vi "Interfaz_Completa.vi"() -> ()   [LabVIEW 2019]
panel:
  out "Datos UART":string
  in  "Nombre .csv":string
  in  "Export Button":bool
  out "UART Error":errorcluster
  out "Valores Tácteles":dbl[][](array[numeric])
  in  "Fila":i32
  in  "Columna":i32
  in  "Selección Modo Datos":T1(ring) caption="Modo Introducción de Datos"
  out "XY Graph":cluster{"Y":dbl[], "Y":dbl[]}[](graph)
  out "Intensity Graph":dbl[][](graph)
  in  "Tab_Introducción_Datos":T2(tab)
  in  "Comando Manual":bool
  in  "Cadena de datos (Manual)":string
  in  "Presión Manual(PSI)":dbl
  in  "Recibir de fichero":bool
  in  "file path (use dialog)":path
  in  "Nº De Ejecuciones":dbl
  in  "Tiempo Entre Medidas(ms)":dbl
  in  "Incremento":dbl
  in  "Presión Min (PSI)":dbl
  in  "Presión Max (PSI)":dbl
  in  "Tiempo Entre Medida(ms)":dbl
  in  "Tiempo Total":dbl
  in  "Presión Deseada (PSI)":dbl
  in  "Histéresis":bool
  in  "Deriva":bool
  in  "Medida Simple":bool
  in  "Tab_Valvula":enum32{"Page 2"}(tab)
  in  "Ejecutar Válvula":bool
  in  "Tipo de Comando":string(combo)
  in  "COM Pneumax":refnum<visa-resource-name>
  in  "Presión Deseada (PSI)":u8 step=5
  in  "Parámetro":u8 step=1
  in  "Valor del Parámetro":u8 max=25 step=1
  out "Presión (PSI)":dbl
  out "Respuesta del regulador":string
  in  "Nombre Nueva Sesión":string
  in  "Tab Control":enum32{"Tab_Automatica", "Tab_Manual"}(tab)
  in  "OK_Automatico":bool
  in  "baud rate PSoC":u32(ring)=9600 items=["75"=75, "110"=110, "134"=134, "150"=150, "300"=300, "600"=600, "1200"=1200, "1800"=1800, "2400"=2400, "4800"=4800, "7200"=7200, "9600"=9600, "14400"=14400, "19200"=19200, "28800"=28800, "38400"=38400, "56000"=56000, "57600"=57600, "115200"=115200, "128000"=128000, "230400"=230400]
  in  "COM PSoC":refnum<visa-resource-name>
  in  "OK_Manual":bool
  in  "NºFilas":i32
  in  "Nº Columnas":i32
  in  "N_Bits":i32
  in  "Proporcional":i32
  in  "Valor_Maximo":i32
  in  "Manual":bool
  in  "Automática":bool
  in  "Plantilla Tácteles":bool[][](array[boolean])
  in  "Home Button":bool
  in  "Sesiones Disponibles":u16(ring) items=["Default", "Prueba1", "Prueba8", "Prueba7", "Manu", "Andres"]
  in  "Stop Button":bool
  in  "Settings Button":bool
  in  "Save Button":bool
  in  "Refresh Button":bool
  in  "Open Button":bool
  # "Fila y Columna del Táctel a Representar"
  # "Abra el fichero que contiene los datos en el formato adecuado y pulse el botón inferior para leer una medida."
  # "Control de Electroválvula Pneumax"
  # "Configure los indicadores del modo Automático. Una vez haya realizado la\nconfiguración, pulse OK."
  # "Configure el número de filas y de columnas, si la medida viene de manera\n proporcional, el Nº de bits que tiene el timer con el que se ha realizado \nla medida y el valor máximo de las medidas. Luego pulse el botón OK y\n coloque los sensores que desee en su plantilla tácteles."
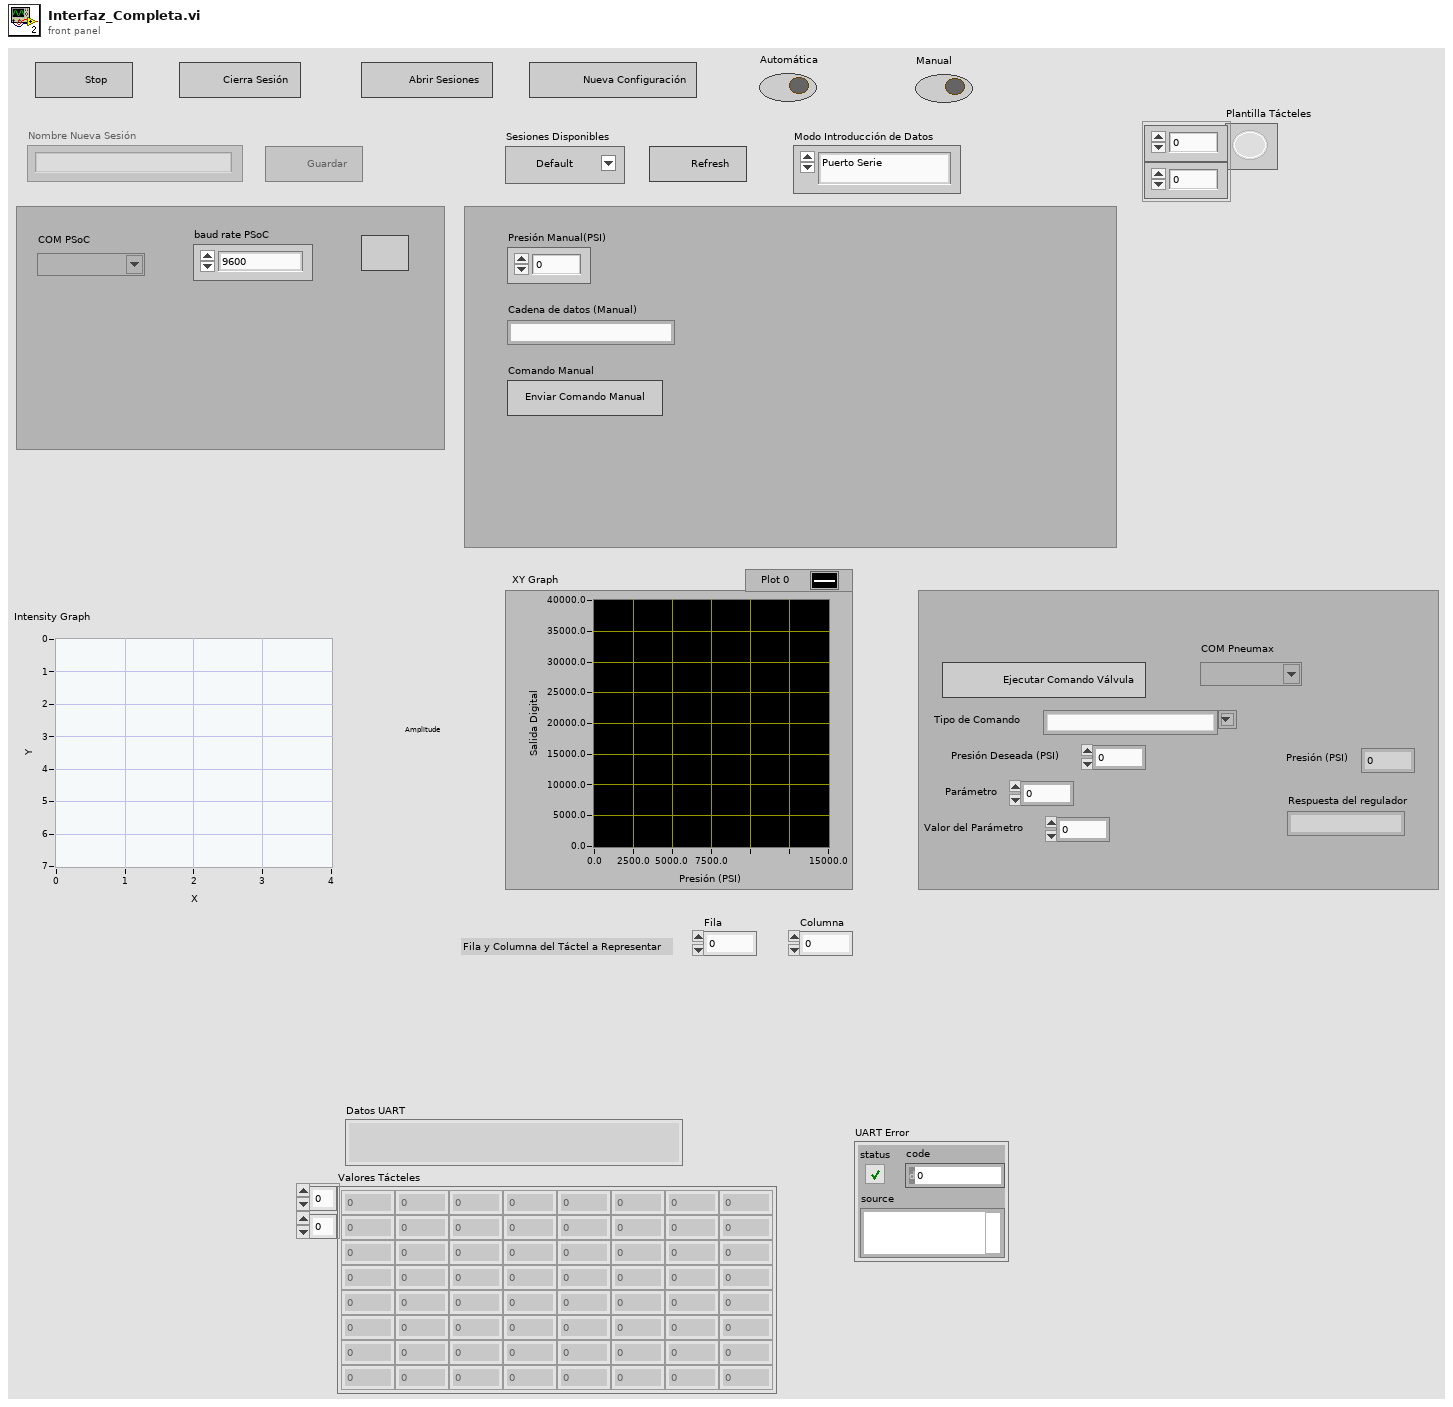
[diagram p1: front panel]
types:
  T1 = enum16{"Puerto Serie", "Archivo Importado", "Manual"}
  T2 = enum32{"Manual", "Archivo Importado", "Puerto Serie"}
  T3 = enum8{"Enabled", "Disabled", "Disabled and Grayed Out"}
  T4 = cluster{"String":string, i32, i32, i32, i32, i32}
  T5 = cluster{"Filas ":i32, "Columnas":i32, "Tacteles_Activados":bool[][]}
  T6 = cluster{"Value":string, "String_Tácteles":string, "Number of Rows":u32, "Number of Columns":u32, "Value":i32, "Value":i32, "Value":i32}
  T7 = cluster{"Value":refnum<visa-resource-name>, "Value":u32, "Value":refnum<visa-resource-name>, "Value":i32, "Value":i32}
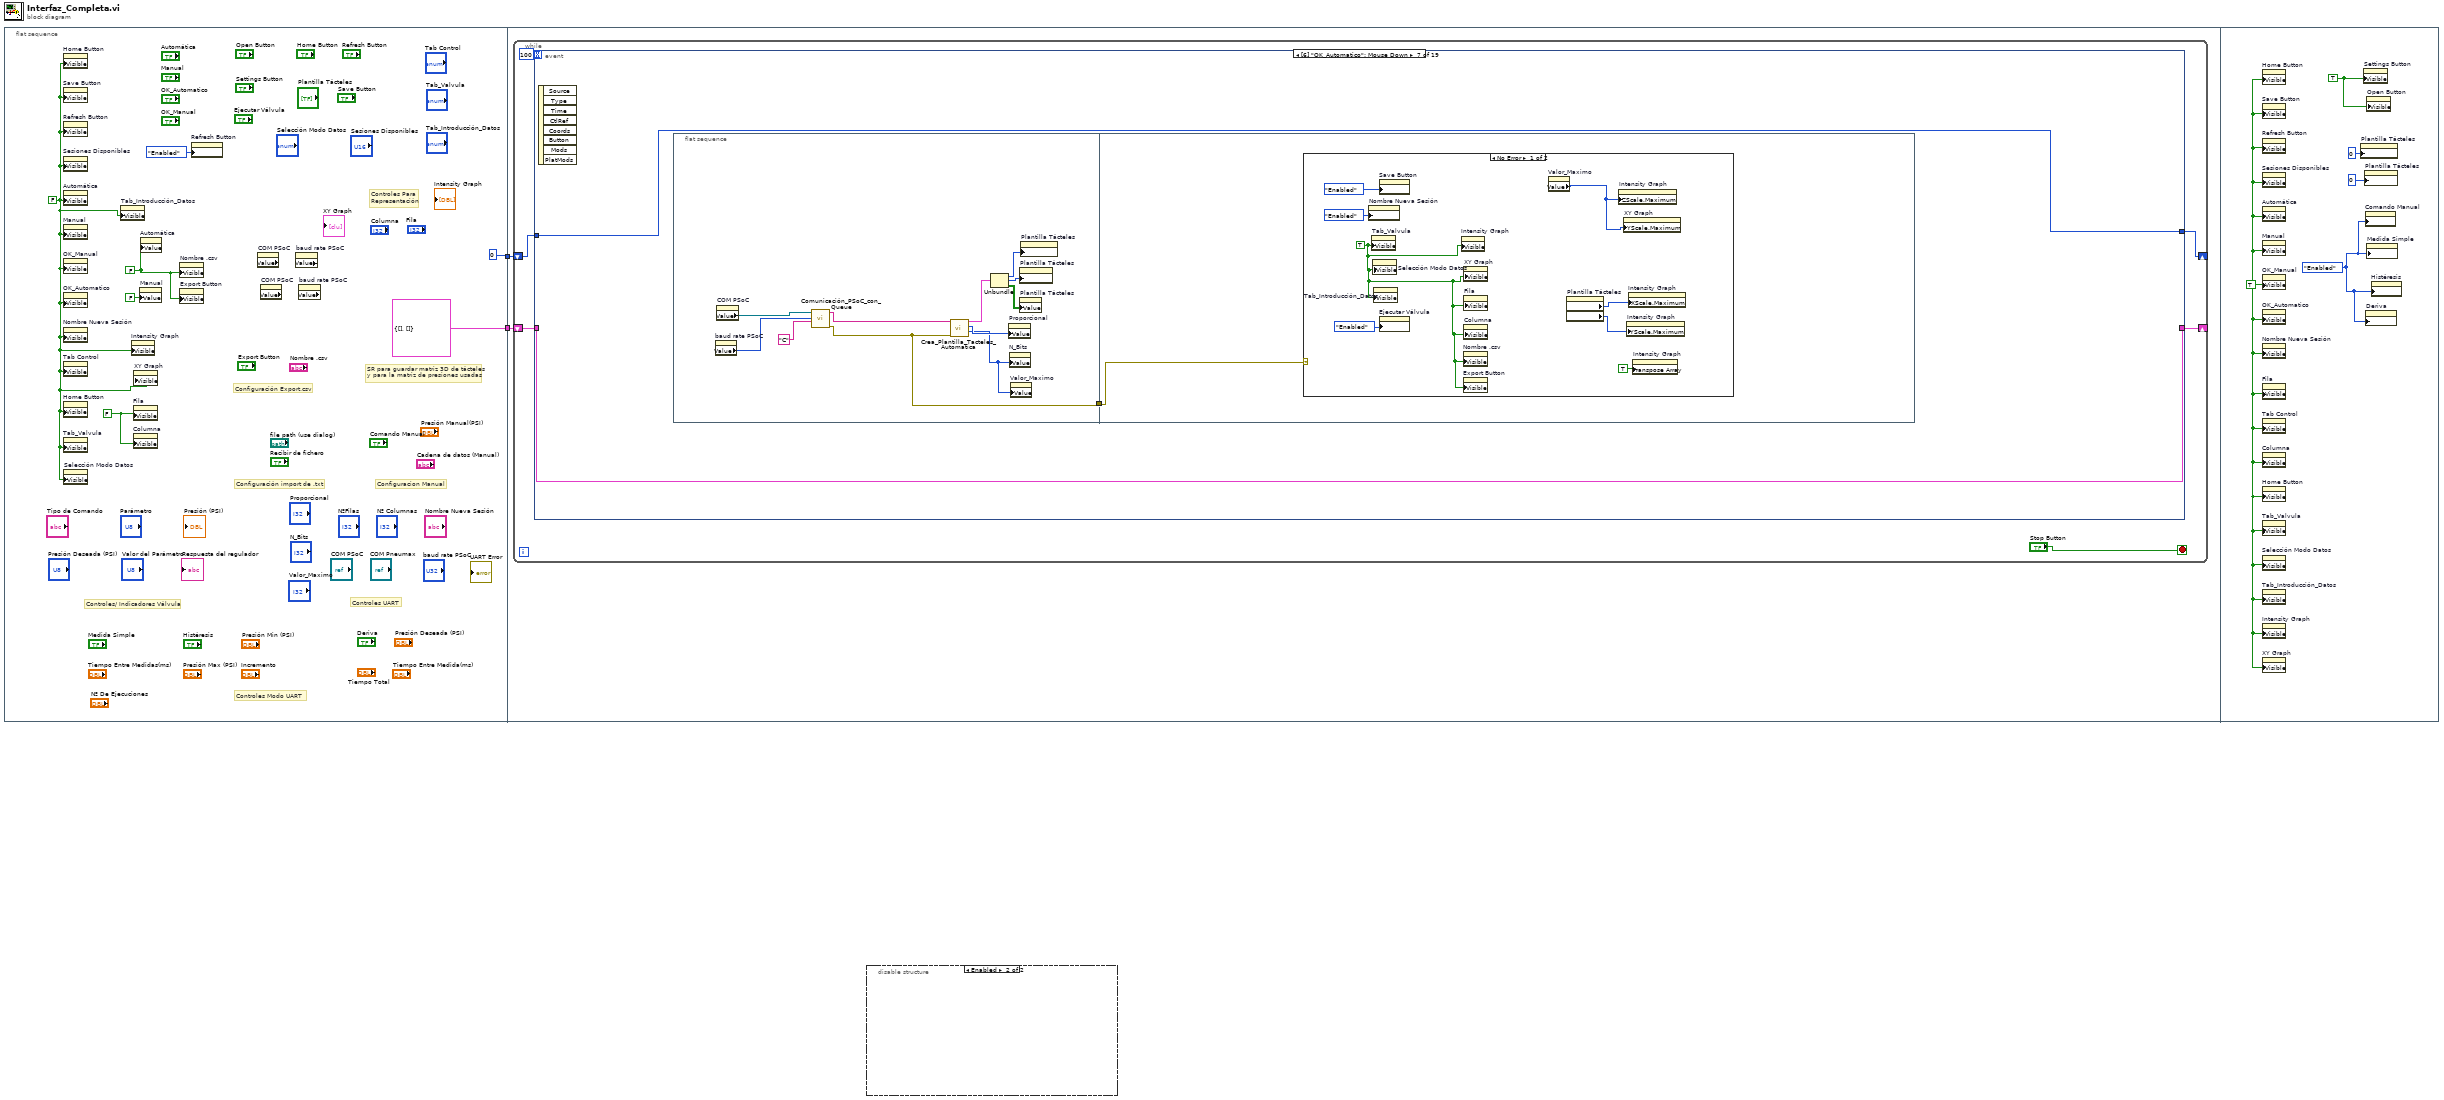
[diagram p0: block diagram]
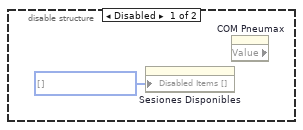
[diagram p2: hidden frame]
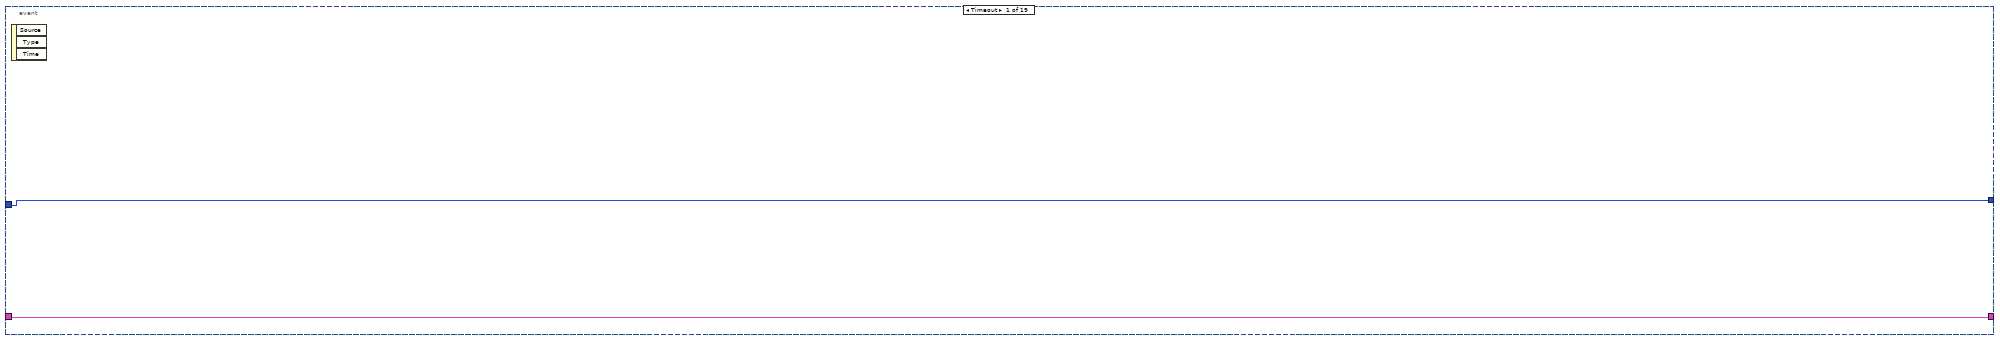
[diagram p3: hidden frame]
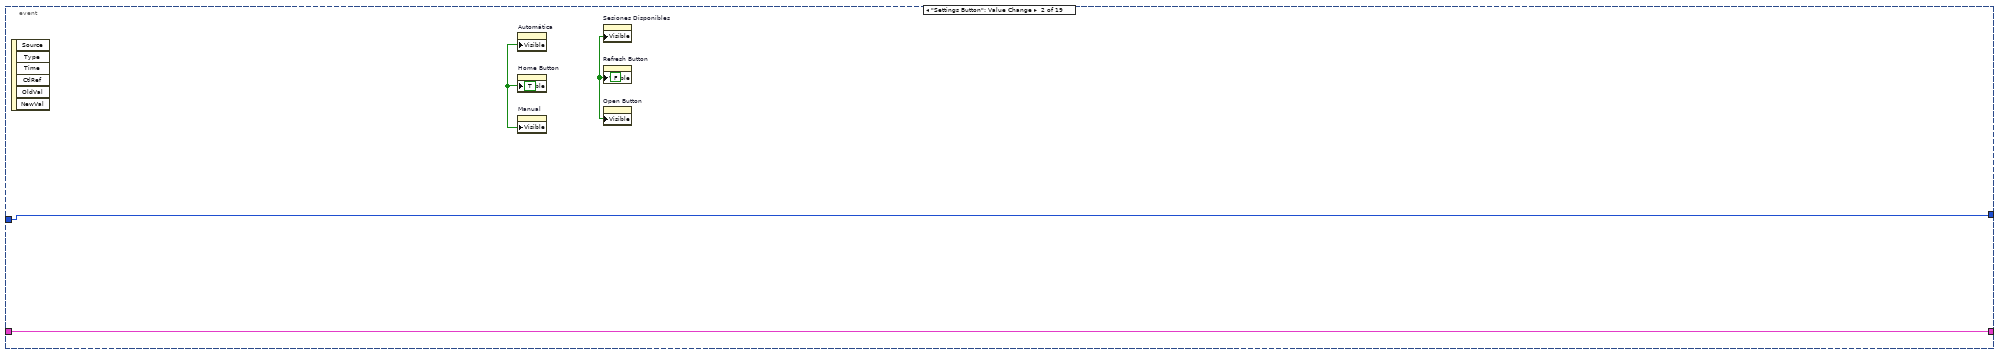
[diagram p4: hidden frame]
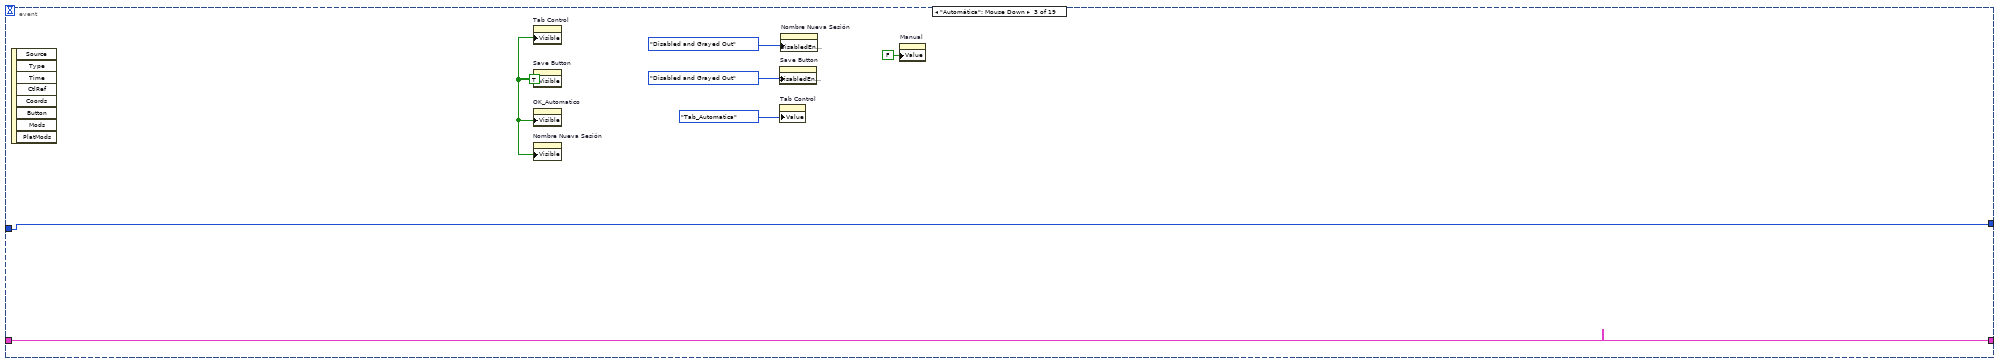
[diagram p5: hidden frame]
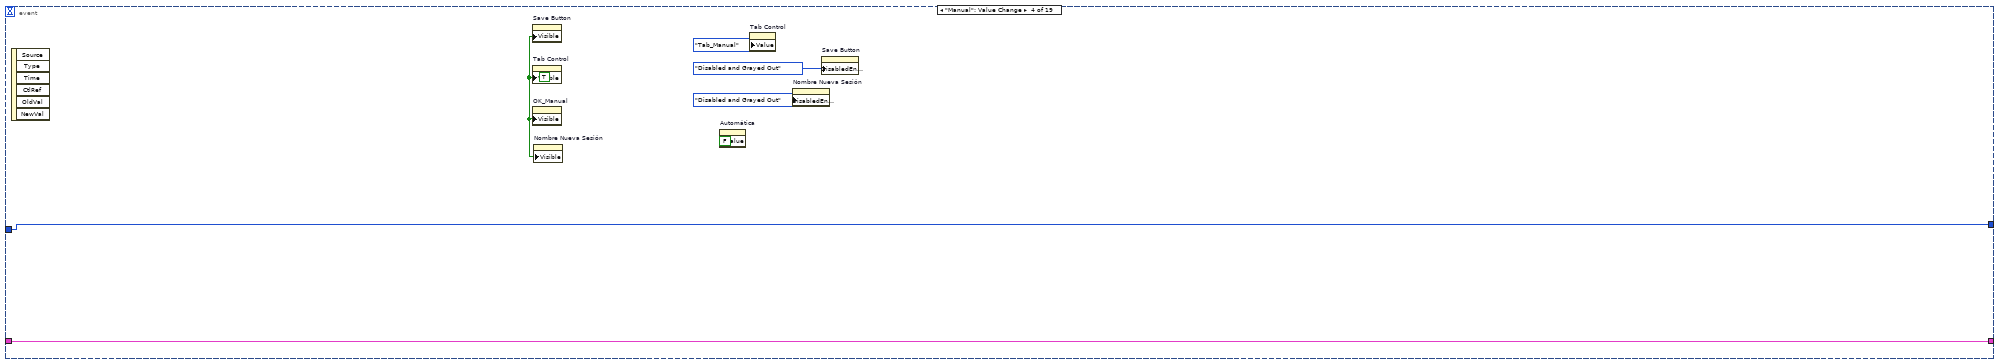
[diagram p6: hidden frame]
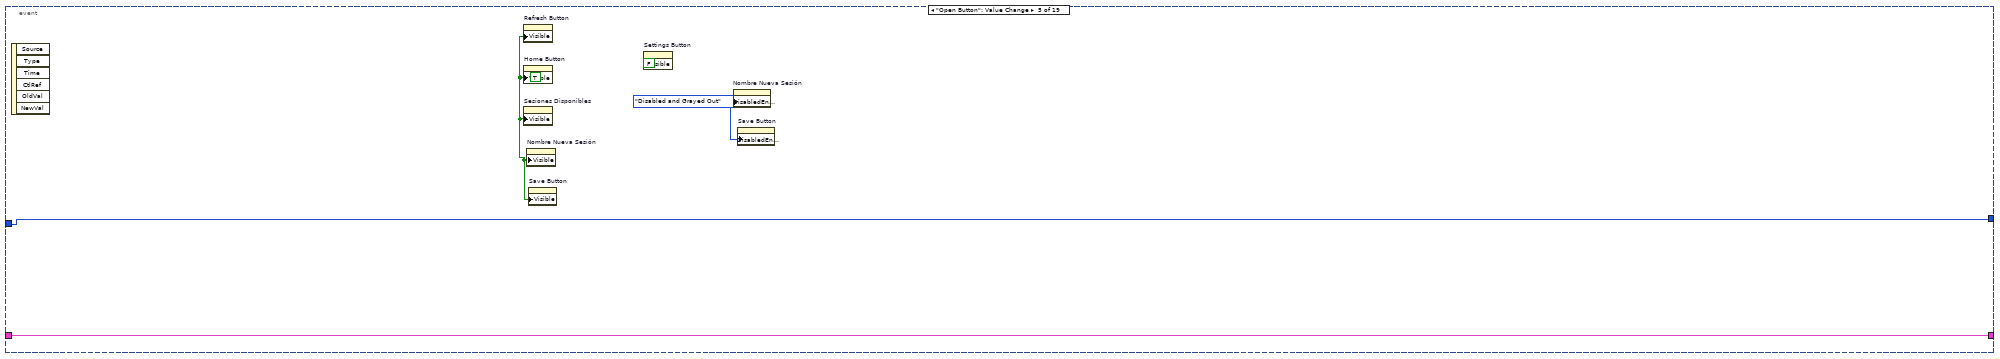
[diagram p7: hidden frame]
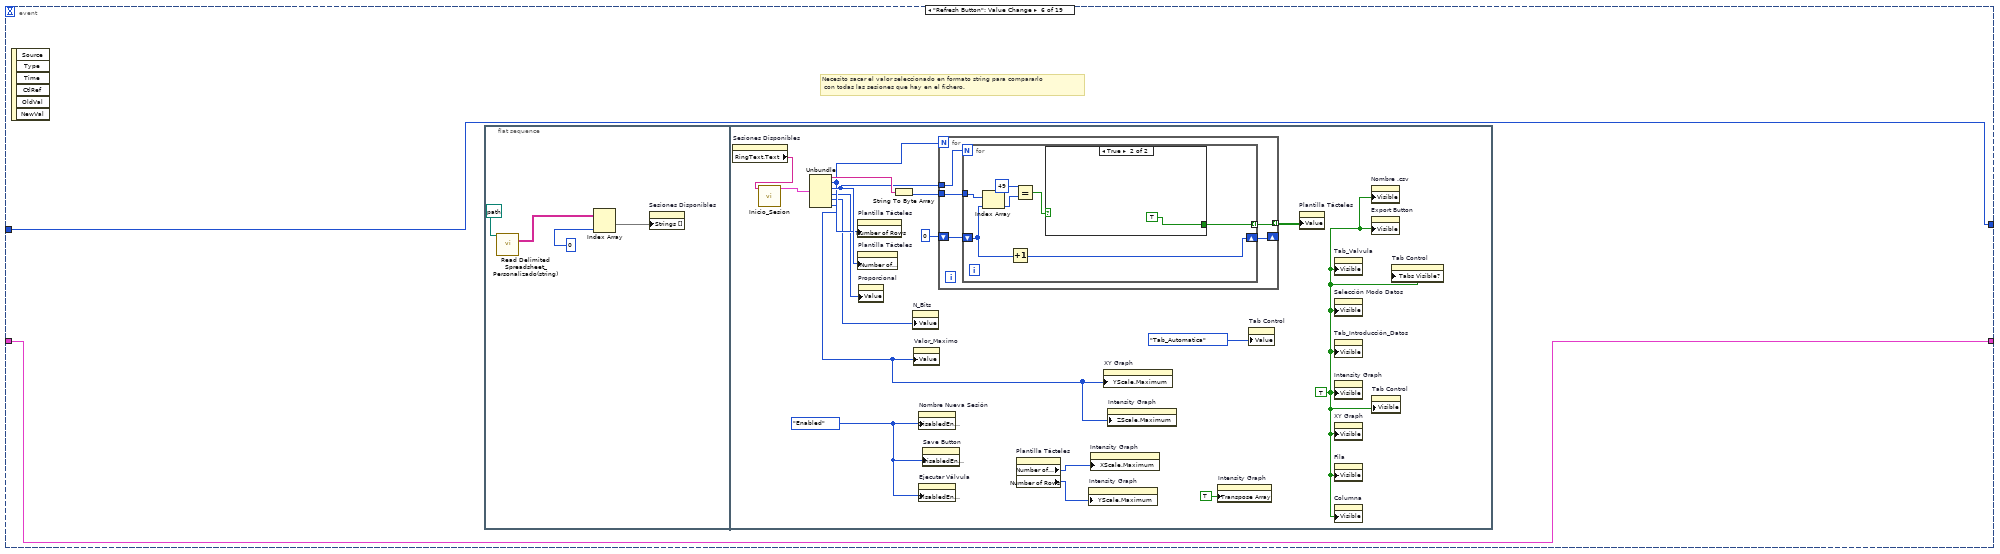
[diagram p8: hidden frame]
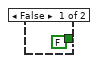
[diagram p9: hidden frame]
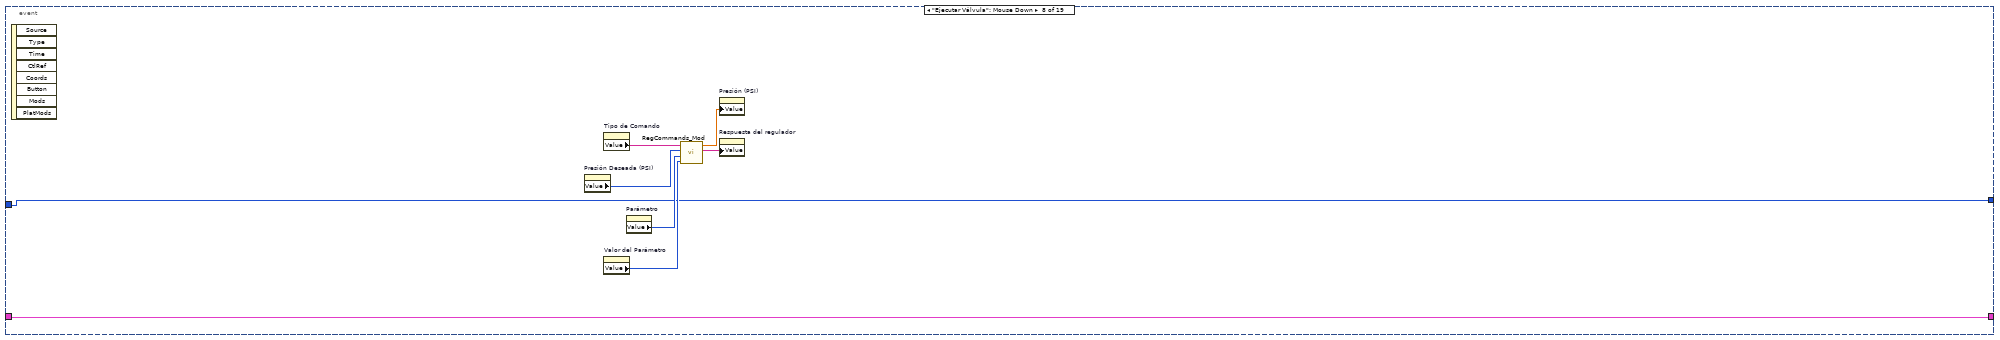
[diagram p11: hidden frame]
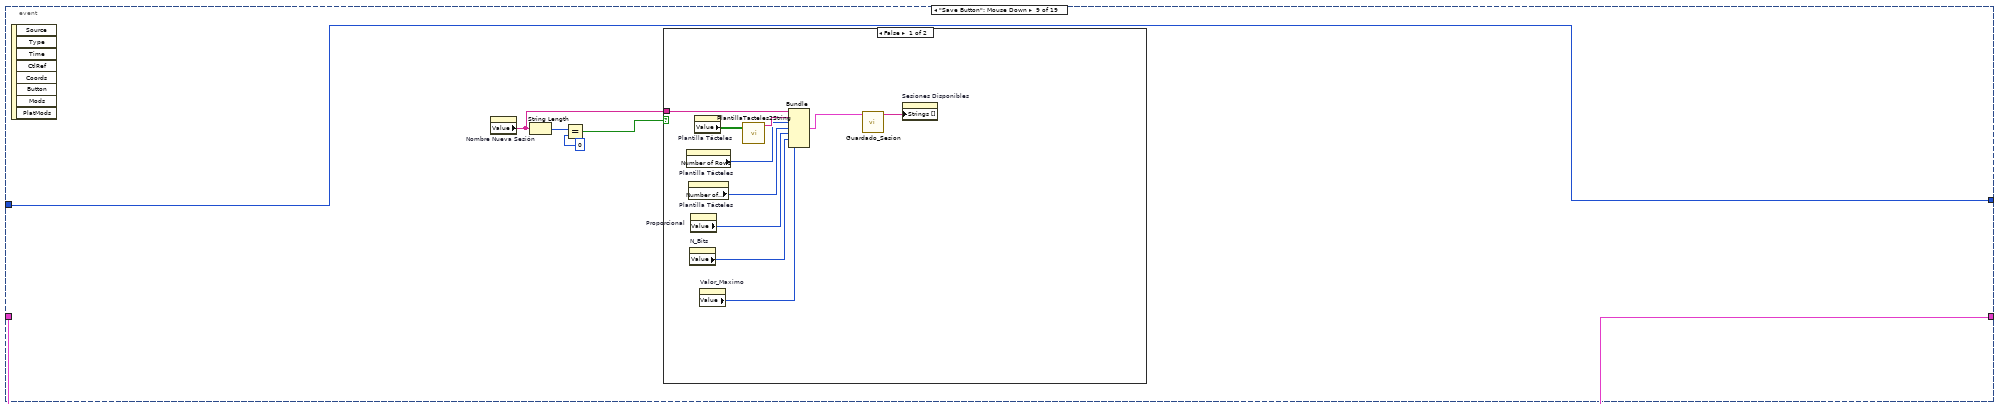
[diagram p12: hidden frame]
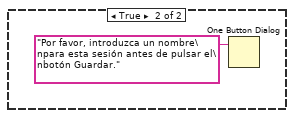
[diagram p13: hidden frame]
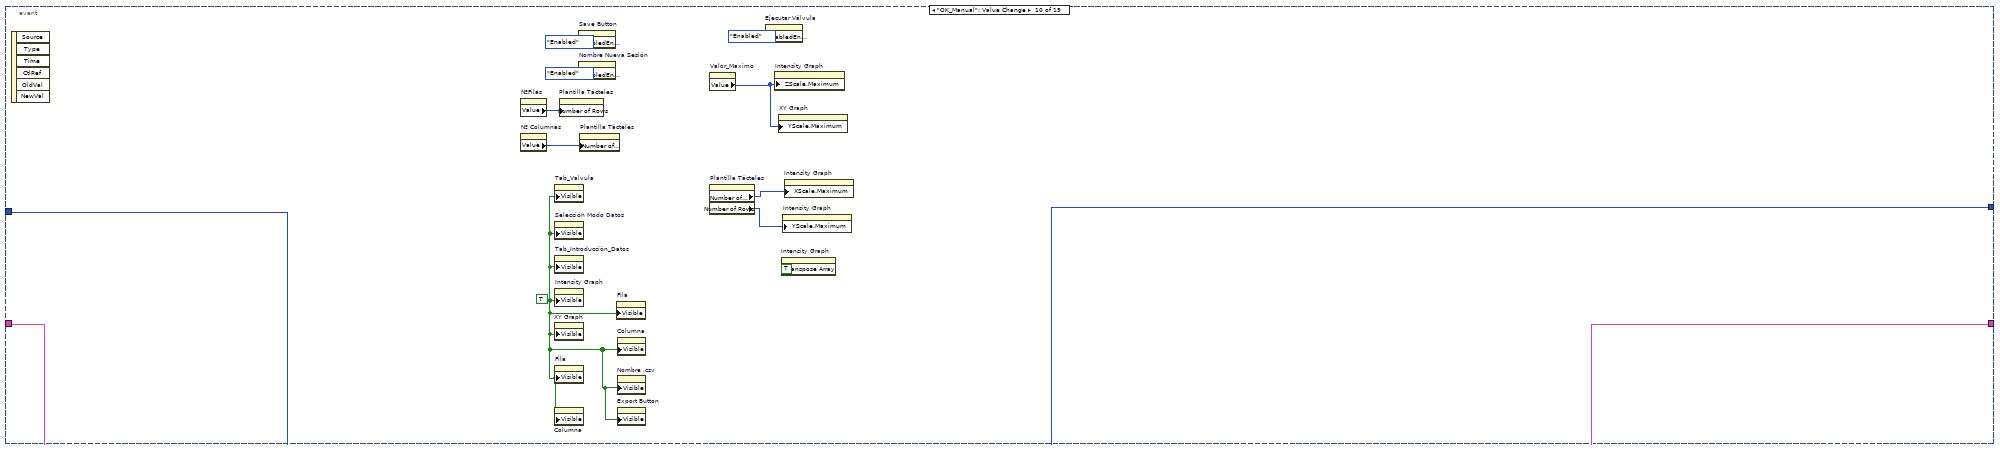
[diagram p14: hidden frame]
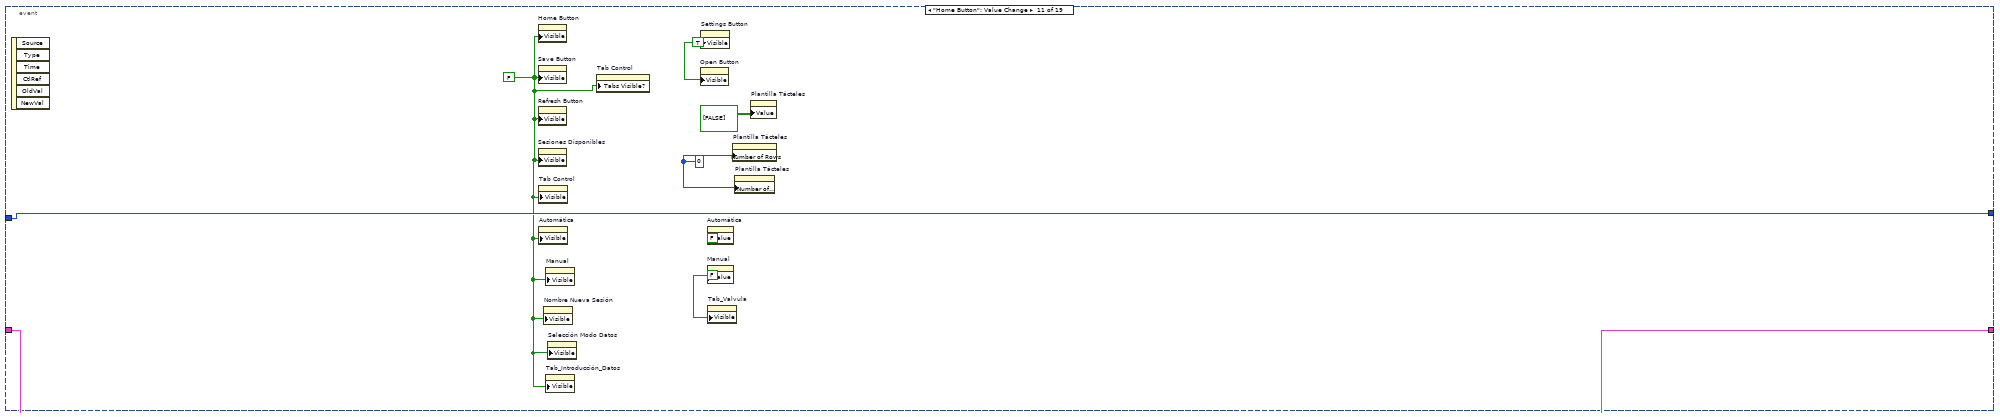
[diagram p15: hidden frame]
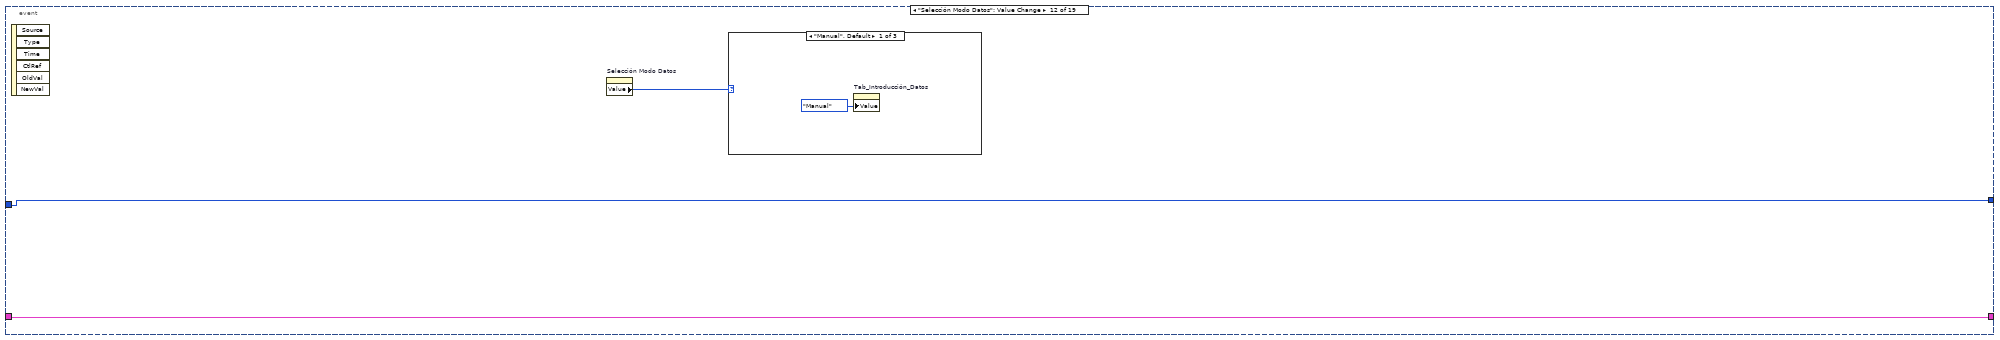
[diagram p16: hidden frame]
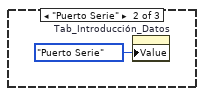
[diagram p17: hidden frame]
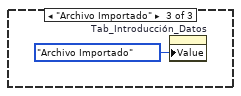
[diagram p18: hidden frame]
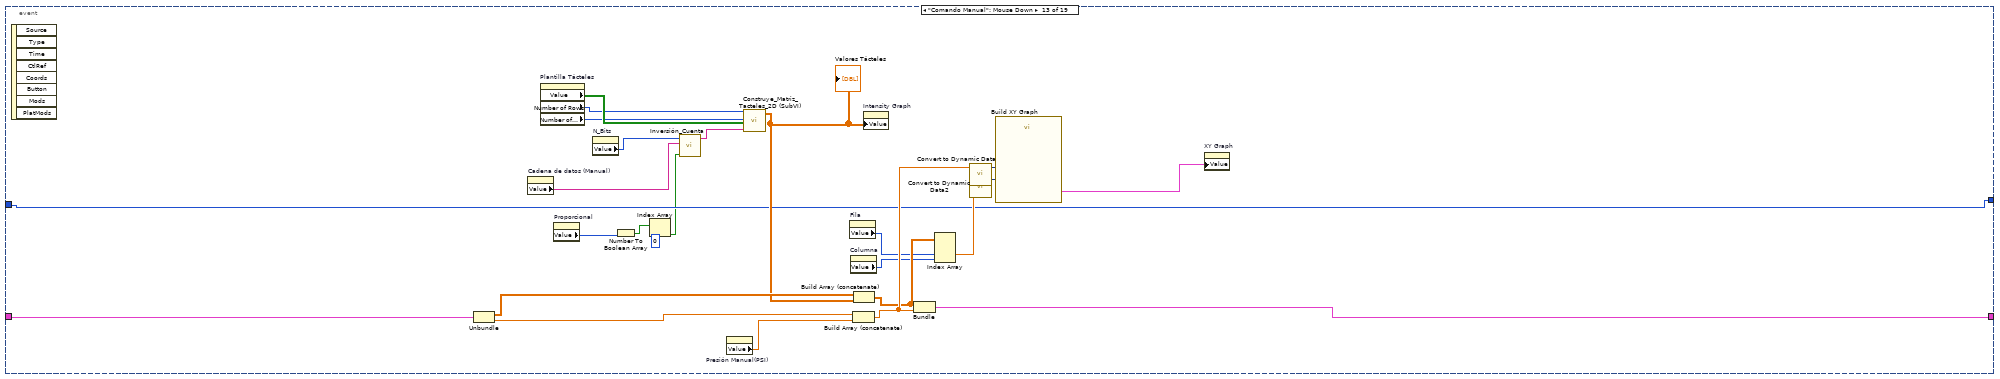
[diagram p19: hidden frame]
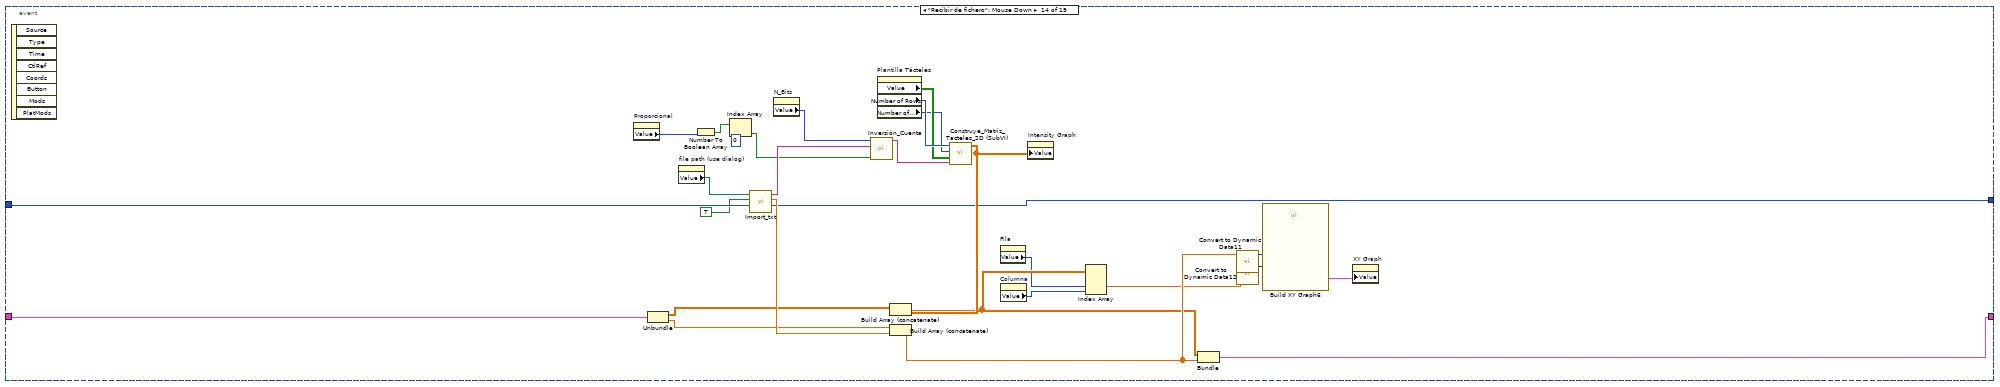
[diagram p20: hidden frame]
diagram:
  n1 = flat-sequence {
    tunnel: [cluster{dbl[][][], dbl[]} {[], []}] -> w2
    tunnel: [0] -> w1
    tunnel: w2 -> [w11]
    tunnel: w1 -> [w10]
    frame #0 {
      w5 = FALSE
      w4 = FALSE ("Automática")
      w6 = FALSE ("Visible")
      # "Configuración Export.csv"
      # "Controles Modo UART"
      # "Configuración import de .txt"
      # "Controles Para \nRepresentación"
      # "SR para guardar matriz 3D de tácteles\ny para la matriz de presiones usadas"
      # "Configuracion Manual"
      # "Controles/ Indicadores Válvula"
      # "Controles UART"
      n2 = property on="Home Button" class="Bool (strict)"("Visible"=w6) -> ()  [unwired: 2 in, 2 out]
      n3 = property on="Save Button" class="Bool (strict)"("Visible"=w6) -> ()  [unwired: 2 in, 2 out]
      n4 = property on="Refresh Button" class="Bool (strict)"("Visible"=w6) -> ()  [unwired: 2 in, 2 out]
      n5 = property on="Sesiones Disponibles" class="Ring (strict)"("Visible"=w6) -> ()  [unwired: 2 in, 2 out]
      n6 = property on="Automática" class="Bool (strict)"("Visible"=w6) -> ()  [unwired: 2 in, 2 out]
      n7 = property on="Manual" class="Bool (strict)"("Visible"=w6) -> ()  [unwired: 2 in, 2 out]
      n8 = property on="OK_Manual" class="Bool (strict)"("Visible"=w6) -> ()  [unwired: 2 in, 2 out]
      n9 = property on="OK_Automatico" class="Bool (strict)"("Visible"=w6) -> ()  [unwired: 2 in, 2 out]
      n10 = property on="Nombre Nueva Sesión" class="Str"("Visible"=w6) -> ()  [unwired: 2 in, 2 out]
      n11 = property on="Tab Control" class="TabCtl (strict)"("Visible"=w6) -> ()  [unwired: 2 in, 2 out]
      n12 = property on="Home Button" class="Bool (strict)"("Visible"=w6) -> ()  [unwired: 2 in, 2 out]
      n13 = property on="Tab_Valvula" class="TabCtl (strict)"("Visible"=w6) -> ()  [unwired: 2 in, 2 out]
      n14 = property on="Selección Modo Datos" class="Enum (strict)"("Visible"=w6) -> ()  [unwired: 2 in, 2 out]
      n15 = property on="Tab_Introducción_Datos" class="TabCtl (strict)"("Visible"=w6) -> ()  [unwired: 2 in, 2 out]
      n16 = property on="Intensity Graph" class="IntGraph (strict)"("Visible"=w6) -> ()  [unwired: 2 in, 2 out]
      n17 = property on="Fila" class="DigNum (strict)"("Visible"=w5) -> ()  [unwired: 2 in, 2 out]
      n18 = property on="Columna" class="DigNum (strict)"("Visible"=w5) -> ()  [unwired: 2 in, 2 out]
      n19 = property on="XY Graph" class="XYGraph (strict)"("Visible"=w6) -> ()  [unwired: 2 in, 2 out]
      n20 = property on="Manual" class="Bool (strict)"("Value"=FALSE ("Manual")) -> ()  [unwired: 2 in, 2 out]
      n21 = property on="Automática" class="Bool (strict)"("Value"=w4) -> ()  [unwired: 2 in, 2 out]
      n22 = property on="Nombre .csv" class="Str"("Visible"=w4) -> ()  [unwired: 2 in, 2 out]
      n23 = property on="Export Button" class="Bool (strict)"("Visible"=w4) -> ()  [unwired: 2 in, 2 out]
      n24 = property on="Refresh Button" class="Bool (strict)"("DisabledEnum"=T3."Enabled" ("Disabled")) -> ()  [unwired: 2 in, 2 out]
      n25 = property on="COM PSoC" class="VISAName" props=["Value"]() -> ()  [unwired: 2 in, 3 out]
      n26 = property on="COM PSoC" class="VISAName" props=["Value"]() -> ()  [unwired: 2 in, 3 out]
      n27 = property on="baud rate PSoC" class="Ring (strict)" props=["Value"]() -> ()  [unwired: 2 in, 3 out]
      n28 = property on="baud rate PSoC" class="Ring (strict)" props=["Value"]() -> ()  [unwired: 2 in, 3 out]
    }
    frame #1 {
      n29 = while {
        shift-right: [w14] -> _
        shift-left: w11 -> [w15]
        shift-right: [w12] -> _
        shift-left: w10 -> [w13]
        stop <- "Stop Button" stop-if-true
        n30 = event shown="[6] \"OK_Automatico\": Mouse Down" {
          selector: _ -> [_ _ _ _ _ _ _ _ _ _ _ _ _ _ _ _ _ _ _]
          dyn-events: _ -> [_ _ _ _ _ _ _ _ _ _ _ _ _ _ _ _ _ _ _]
          timeout: 100 -> [_ _ _ _ _ _ _ _ _ _ _ _ _ _ _ _ _ _ _]
          tunnel: w15 -> [w19 w21 w25 w32 w39 w44 w82 w104 w112 w132 w142 w149 w175 w205 w238 w248 w295 w366 _]
          tunnel: [w19 w21 w25 w32 w39 w44 w82 w104 w112 w132 w142 w149 w171 w189 w223 w243 w292 w365 _] -> w14
          tunnel: w13 -> [w18 w20 w24 w31 w38 w43 w80 w103 w111 w129 w141 w148 w161 w188 w215 w240 w291 w364 w378]
          tunnel: [w18 w20 w24 w31 w38 w43 w80 w103 w111 w129 w141 w148 w161 w187 w215 w240 w291 w364 w378] -> w12
          event Timeout {
            n31 = event-data() -> ()  [unwired: 1 in, 3 out]
          }
          event "Settings Button": Value Change {
            w22 = FALSE ("Automática")
            w23 = TRUE ("Automática")
            n32 = event-data() -> ()  [unwired: 1 in, 6 out]
            n33 = property on="Automática" class="Bool (strict)"("Visible"=w23) -> ()  [unwired: 2 in, 2 out]
            n34 = property on="Home Button" class="Bool (strict)"("Visible"=w23) -> ()  [unwired: 2 in, 2 out]
            n35 = property on="Manual" class="Bool (strict)"("Visible"=w23) -> ()  [unwired: 2 in, 2 out]
            n36 = property on="Sesiones Disponibles" class="Ring (strict)"("Visible"=w22) -> ()  [unwired: 2 in, 2 out]
            n37 = property on="Refresh Button" class="Bool (strict)"("Visible"=w22) -> ()  [unwired: 2 in, 2 out]
            n38 = property on="Open Button" class="Bool (strict)"("Visible"=w22) -> ()  [unwired: 2 in, 2 out]
          }
          event "Automática": Mouse Down {
            w27 = TRUE ("Visible")
            n39 = event-data() -> ()  [unwired: 1 in, 8 out]
            n40 = property on="Tab Control" class="TabCtl (strict)"("Visible"=w27) -> ()  [unwired: 2 in, 2 out]
            n41 = property on="Save Button" class="Bool (strict)"("Visible"=w27) -> ()  [unwired: 2 in, 2 out]
            n42 = property on="OK_Automatico" class="Bool (strict)"("Visible"=w27) -> ()  [unwired: 2 in, 2 out]
            n43 = property on="Nombre Nueva Sesión" class="Str"("Visible"=w27) -> ()  [unwired: 2 in, 2 out]
            n44 = property on="Save Button" class="Bool (strict)"("DisabledEnum"=T3."Disabled and Grayed Out" ("Disabled")) -> ()  [unwired: 2 in, 2 out]
            n45 = property on="Tab Control" class="TabCtl (strict)"("Value"=enum32{"Tab_Automatica", "Tab_Manual"}."Tab_Automatica" ("Tab Control")) -> ()  [unwired: 2 in, 2 out]
            n46 = property on="Nombre Nueva Sesión" class="Str"("DisabledEnum"=T3."Disabled and Grayed Out" ("Disabled")) -> ()  [unwired: 2 in, 2 out]
            n47 = property on="Manual" class="Bool (strict)"("Value"=FALSE ("Manual")) -> ()  [unwired: 2 in, 2 out]
          }
          event "Manual": Value Change {
            w35 = TRUE
            n48 = event-data() -> ()  [unwired: 1 in, 6 out]
            n49 = property on="Save Button" class="Bool (strict)"("Visible"=w35) -> ()  [unwired: 2 in, 2 out]
            n50 = property on="Tab Control" class="TabCtl (strict)"("Visible"=w35) -> ()  [unwired: 2 in, 2 out]
            n51 = property on="OK_Manual" class="Bool (strict)"("Visible"=w35) -> ()  [unwired: 2 in, 2 out]
            n52 = property on="Nombre Nueva Sesión" class="Str"("Visible"=w35) -> ()  [unwired: 2 in, 2 out]
            n53 = property on="Automática" class="Bool (strict)"("Value"=FALSE ("Automática")) -> ()  [unwired: 2 in, 2 out]
            n54 = property on="Tab Control" class="TabCtl (strict)"("Value"=enum32{"Tab_Automatica", "Tab_Manual"}."Tab_Manual" ("Tab Control")) -> ()  [unwired: 2 in, 2 out]
            n55 = property on="Nombre Nueva Sesión" class="Str"("DisabledEnum"=T3."Disabled and Grayed Out" ("Disabled")) -> ()  [unwired: 2 in, 2 out]
            n56 = property on="Save Button" class="Bool (strict)"("DisabledEnum"=T3."Disabled and Grayed Out" ("Disabled")) -> ()  [unwired: 2 in, 2 out]
          }
          event "Open Button": Value Change {
            w40 = T3."Disabled and Grayed Out" ("Disabled")
            w41 = TRUE ("Visible")
            n57 = event-data() -> ()  [unwired: 1 in, 6 out]
            n58 = property on="Refresh Button" class="Bool (strict)"("Visible"=w41) -> ()  [unwired: 2 in, 2 out]
            n59 = property on="Home Button" class="Bool (strict)"("Visible"=w41) -> ()  [unwired: 2 in, 2 out]
            n60 = property on="Sesiones Disponibles" class="Ring (strict)"("Visible"=w41) -> ()  [unwired: 2 in, 2 out]
            n61 = property on="Nombre Nueva Sesión" class="Str"("Visible"=w41) -> ()  [unwired: 2 in, 2 out]
            n62 = property on="Save Button" class="Bool (strict)"("Visible"=w41) -> ()  [unwired: 2 in, 2 out]
            n63 = property on="Settings Button" class="Bool (strict)"("Visible"=FALSE) -> ()  [unwired: 2 in, 2 out]
            n64 = property on="Nombre Nueva Sesión" class="Str"("DisabledEnum"=w40) -> ()  [unwired: 2 in, 2 out]
            n65 = property on="Save Button" class="Bool (strict)"("DisabledEnum"=w40) -> ()  [unwired: 2 in, 2 out]
          }
          event "Refresh Button": Value Change {
            # "Necesito sacar el valor seleccionado en formato string para compararlo\n con todas las sesiones que hay en el fichero."
            n66 = event-data() -> ()  [unwired: 1 in, 6 out]
            n67 = flat-sequence {
              frame #0 {
                n68 = call "Read Delimited Spreadsheet_Personalizado(string).vi"("file path (dialog if empty)"=path "C:/Users/manu_/OneDrive/Escritorio/Universidad/24-25/2ºCuatri/Trabajo Fin Grado/LabVIEW/Sesiones/Configuraciones.txt" ("file path (use dialog)")) -> ("all rows"=w45:string[][])  [unwired: 9 in, 5 out]
                n69 = Index Array(array=w45, index (col)=0 ("disabled index (col)")) -> (element=w47:string[])  [unwired: 1 in]
                n70 = property on="Sesiones Disponibles" class="Ring (strict)"("Strings []"=w47) -> ()  [unwired: 2 in, 2 out]
              }
              frame #1 {
                w58 = T3."Enabled" ("Disabled")
                w49 = TRUE ("Visible")
                n71 = property on="Sesiones Disponibles" class="Ring (strict)"() -> ("RingText.Text"=w65:string)  [unwired: 2 in, 2 out]
                n72 = call "Inicio_Sesion.vi"("Sesion_Requerida"=w65) -> ("Configuracion_Out"=w64:T4)  [unwired: 10 in]
                n73 = Unbundle(w64) -> ("String"=w63:string, w57:i32, w59:i32, w56:i32, w55:i32, w51:i32)
                n74 = property on="Plantilla Tácteles" class="Arr (strict)"("Number of Rows"=w57) -> ()  [unwired: 2 in, 2 out]
                n75 = property on="Plantilla Tácteles" class="Arr (strict)"("Number of Columns"=w59) -> ()  [unwired: 2 in, 2 out]
                n76 = property on="Proporcional" class="DigNum (strict)"("Value"=w56) -> ()  [unwired: 2 in, 2 out]
                n77 = String To Byte Array(string=w63) -> (unsigned byte array=w62:u8[])
                n78 = property on="N_Bits" class="DigNum (strict)"("Value"=w55) -> ()  [unwired: 2 in, 2 out]
                n79 = property on="Valor_Maximo" class="DigNum (strict)"("Value"=w51) -> ()  [unwired: 2 in, 2 out]
                n80 = property on="Nombre Nueva Sesión" class="Str"("DisabledEnum"=w58) -> ()  [unwired: 2 in, 2 out]
                n81 = property on="Ejecutar Válvula" class="Bool (strict)"("DisabledEnum"=w58) -> ()  [unwired: 2 in, 2 out]
                n82 = property on="Save Button" class="Bool (strict)"("DisabledEnum"=w58) -> ()  [unwired: 2 in, 2 out]
                n83 = for {
                  N: w57 -> [_]
                  tunnel: w62 -> [w70]
                  shift-right: [w68] -> _
                  shift-left: 0 -> [w69]
                  tunnel: [w67] -> w60 mode=indexing
                  tunnel: w59 -> [w66]
                  n84 = for {
                    N: w66 -> [_]
                    tunnel: w70 -> [w77]
                    shift-right: [w72] -> w68
                    shift-left: w69 -> [w73]
                    tunnel: [w71] -> w67 mode=indexing
                    n85 = Index Array(array=w77, index=w73) -> (element=w76:u8)
                    n86 = Increment(x=w73) -> (x+1=w72:i32)
                    n87 = Equal?(x=u8 49, y=w76) -> (x = y?=w74:bool)
                    n88 = case shown="True" w74 {
                      tunnel: [FALSE TRUE] -> w71
                      frame False {
                      }
                      frame True {
                      }
                    }
                  }
                }
                n89 = property on="Plantilla Tácteles" class="Arr (strict)"() -> ("Number of Columns"=w53:u32, "Number of Rows"=w52:u32)  [unwired: 2 in, 2 out]
                n90 = property on="Intensity Graph" class="IntGraph (strict)"("YScale.Maximum"=w52) -> ()  [unwired: 2 in, 2 out]
                n91 = property on="Intensity Graph" class="IntGraph (strict)"("XScale.Maximum"=w53) -> ()  [unwired: 2 in, 2 out]
                n92 = property on="XY Graph" class="XYGraph (strict)"("YScale.Maximum"=w51) -> ()  [unwired: 2 in, 2 out]
                n93 = property on="Intensity Graph" class="IntGraph (strict)"("ZScale.Maximum"=w51) -> ()  [unwired: 2 in, 2 out]
                n94 = property on="Intensity Graph" class="IntGraph (strict)"("Transpose Array"=TRUE) -> ()  [unwired: 2 in, 2 out]
                n95 = property on="Tab Control" class="TabCtl (strict)"("Value"=enum32{"Tab_Automatica", "Tab_Manual"}."Tab_Automatica" ("Tab Control")) -> ()  [unwired: 2 in, 2 out]
                n96 = property on="Plantilla Tácteles" class="Arr (strict)"("Value"=w60) -> ()  [unwired: 2 in, 2 out]
                n97 = property on="Tab_Valvula" class="TabCtl (strict)"("Visible"=w49) -> ()  [unwired: 2 in, 2 out]
                n98 = property on="Selección Modo Datos" class="Enum (strict)"("Visible"=w49) -> ()  [unwired: 2 in, 2 out]
                n99 = property on="Tab_Introducción_Datos" class="TabCtl (strict)"("Visible"=w49) -> ()  [unwired: 2 in, 2 out]
                n100 = property on="Intensity Graph" class="IntGraph (strict)"("Visible"=w49) -> ()  [unwired: 2 in, 2 out]
                n101 = property on="XY Graph" class="XYGraph (strict)"("Visible"=w49) -> ()  [unwired: 2 in, 2 out]
                n102 = property on="Fila" class="DigNum (strict)"("Visible"=w49) -> ()  [unwired: 2 in, 2 out]
                n103 = property on="Columna" class="DigNum (strict)"("Visible"=w49) -> ()  [unwired: 2 in, 2 out]
                n104 = property on="Nombre .csv" class="Str"("Visible"=w49) -> ()  [unwired: 2 in, 2 out]
                n105 = property on="Export Button" class="Bool (strict)"("Visible"=w49) -> ()  [unwired: 2 in, 2 out]
                n106 = property on="Tab Control" class="TabCtl (strict)"("Visible"=w49) -> ()  [unwired: 2 in, 2 out]
                n107 = property on="Tab Control" class="TabCtl (strict)"("Tabs Visible?"=w49) -> ()  [unwired: 2 in, 2 out]
              }
            }
          }
          event "OK_Automatico": Mouse Down {
            n108 = event-data() -> ()  [unwired: 1 in, 8 out]
            n109 = flat-sequence {
              tunnel: [w86] -> w81
              tunnel: w81 -> [w94]
              frame #0 {
                n110 = property on="baud rate PSoC" class="Ring (strict)"() -> ("Value"=w88:u32)  [unwired: 2 in, 2 out]
                n111 = property on="COM PSoC" class="VISAName"() -> ("Value"=w89:refnum<visa-resource-name>)  [unwired: 2 in, 2 out]
                n112 = call "Comunicación_PSoC_con_Queue.vi"("write buffer"="C", "baud rate"=w88, "VISA resource name"=w89) -> ("UART Error"=w86:errorcluster, "String Salida"=w85:string)  [unwired: 6 in, 1 out]
                n113 = call "Crea_Plantilla_Tacteles_Automatica.vi"("error UART"=w86, "Configuración Entrada"=w85) -> ("N_Bits"=w83:i32, "Proporcional"=w84:i32, "Matriz_Configuracion"=w93:T5)  [unwired: 6 in, 1 out]
                n114 = Unbundle(w93) -> ("Filas"=w92:i32, "Columnas"=w91:i32, "Tacteles_Activados"=w90:bool[][])
                n115 = property on="Proporcional" class="DigNum (strict)"("Value"=w84) -> ()  [unwired: 2 in, 2 out]
                n116 = property on="N_Bits" class="DigNum (strict)"("Value"=w83) -> ()  [unwired: 2 in, 2 out]
                n117 = property on="Valor_Maximo" class="DigNum (strict)"("Value"=w83) -> ()  [unwired: 2 in, 2 out]
                n118 = property on="Plantilla Tácteles" class="Arr (strict)"("Number of Columns"=w91) -> ()  [unwired: 2 in, 2 out]
                n119 = property on="Plantilla Tácteles" class="Arr (strict)"("Value"=w90) -> ()  [unwired: 2 in, 2 out]
                n120 = property on="Plantilla Tácteles" class="Arr (strict)"("Number of Rows"=w92) -> ()  [unwired: 2 in, 2 out]
              }
              frame #1 {
                n121 = case shown="No Error" w94 {
                  frame No Error {
                    w96 = TRUE ("Visible")
                    n122 = property on="Nombre Nueva Sesión" class="Str"("DisabledEnum"=T3."Enabled" ("Disabled")) -> ()  [unwired: 2 in, 2 out]
                    n123 = property on="Tab_Valvula" class="TabCtl (strict)"("Visible"=w96) -> ()  [unwired: 2 in, 2 out]
                    n124 = property on="Selección Modo Datos" class="Enum (strict)"("Visible"=w96) -> ()  [unwired: 2 in, 2 out]
                    n125 = property on="Tab_Introducción_Datos" class="TabCtl (strict)"("Visible"=w96) -> ()  [unwired: 2 in, 2 out]
                    n126 = property on="Save Button" class="Bool (strict)"("DisabledEnum"=T3."Enabled" ("Disabled")) -> ()  [unwired: 2 in, 2 out]
                    n127 = property on="Ejecutar Válvula" class="Bool (strict)"("DisabledEnum"=T3."Enabled" ("Disabled")) -> ()  [unwired: 2 in, 2 out]
                    n128 = property on="Intensity Graph" class="IntGraph (strict)"("Visible"=w96) -> ()  [unwired: 2 in, 2 out]
                    n129 = property on="Nombre .csv" class="Str"("Visible"=w96) -> ()  [unwired: 2 in, 2 out]
                    n130 = property on="Export Button" class="Bool (strict)"("Visible"=w96) -> ()  [unwired: 2 in, 2 out]
                    n131 = property on="XY Graph" class="XYGraph (strict)"("Visible"=w96) -> ()  [unwired: 2 in, 2 out]
                    n132 = property on="Fila" class="DigNum (strict)"("Visible"=w96) -> ()  [unwired: 2 in, 2 out]
                    n133 = property on="Columna" class="DigNum (strict)"("Visible"=w96) -> ()  [unwired: 2 in, 2 out]
                    n134 = property on="Valor_Maximo" class="DigNum (strict)"() -> ("Value"=w95:i32)  [unwired: 2 in, 2 out]
                    n135 = property on="Plantilla Tácteles" class="Arr (strict)"() -> ("Number of Columns"=w99:u32, "Number of Rows"=w98:u32)  [unwired: 2 in, 2 out]
                    n136 = property on="Intensity Graph" class="IntGraph (strict)"("ZScale.Maximum"=w95) -> ()  [unwired: 2 in, 2 out]
                    n137 = property on="XY Graph" class="XYGraph (strict)"("YScale.Maximum"=w95) -> ()  [unwired: 2 in, 2 out]
                    n138 = property on="Intensity Graph" class="IntGraph (strict)"("YScale.Maximum"=w98) -> ()  [unwired: 2 in, 2 out]
                    n139 = property on="Intensity Graph" class="IntGraph (strict)"("XScale.Maximum"=w99) -> ()  [unwired: 2 in, 2 out]
                    n140 = property on="Intensity Graph" class="IntGraph (strict)"("Transpose Array"=TRUE) -> ()  [unwired: 2 in, 2 out]
                  }
                  frame Error {
                  }
                }
              }
            }
          }
          event "Ejecutar Válvula": Mouse Down {
            n141 = event-data() -> ()  [unwired: 1 in, 8 out]
            n142 = property on="Presión Deseada (PSI)" class="DigNum (strict)"() -> ("Value"=w105:u8)  [unwired: 2 in, 2 out]
            n143 = property on="Tipo de Comando" class="CmbBox"() -> ("Value"=w108:string)  [unwired: 2 in, 2 out]
            n144 = property on="Valor del Parámetro" class="DigNum (strict)"() -> ("Value"=w107:u8)  [unwired: 2 in, 2 out]
            n145 = property on="Parámetro" class="DigNum (strict)"() -> ("Value"=w106:u8)  [unwired: 2 in, 2 out]
            n146 = call "RegCommands_Mod.vi"("Parameter value"=w107, "Parameter"=w106, "Desired pressure (PSI)"=w105, "Command Type"=w108) -> ("Regulator answer"=w110:string, "Pressure (PSI)"=w109:dbl)  [unwired: 6 in]
            n147 = property on="Presión (PSI)" class="DigNum (strict)"("Value"=w109) -> ()  [unwired: 2 in, 2 out]
            n148 = property on="Respuesta del regulador" class="Str"("Value"=w110) -> ()  [unwired: 2 in, 2 out]
          }
          event "Save Button": Mouse Down {
            n149 = event-data() -> ()  [unwired: 1 in, 8 out]
            n150 = property on="Nombre Nueva Sesión" class="Str"() -> ("Value"=w113:string)  [unwired: 2 in, 2 out]
            n151 = String Length(string=w113) -> (length=w116:i32)
            n152 = Equal?(x=w116, y=0) -> (x = y?=w114:bool)
            n153 = case shown="False" w114 {
              tunnel: w113 -> [w125 _]
              frame False {
                n154 = property on="Plantilla Tácteles" class="Arr (strict)"() -> ("Number of Rows"=w122:u32)  [unwired: 2 in, 2 out]
                n155 = property on="Plantilla Tácteles" class="Arr (strict)"() -> ("Number of Columns"=w119:u32)  [unwired: 2 in, 2 out]
                n156 = property on="N_Bits" class="DigNum (strict)"() -> ("Value"=w120:i32)  [unwired: 2 in, 2 out]
                n157 = property on="Proporcional" class="DigNum (strict)"() -> ("Value"=w121:i32)  [unwired: 2 in, 2 out]
                n158 = property on="Plantilla Tácteles" class="Arr (strict)"() -> ("Value"=w124:bool[][])  [unwired: 2 in, 2 out]
                n159 = property on="Valor_Maximo" class="DigNum (strict)"() -> ("Value"=w117:i32)  [unwired: 2 in, 2 out]
                n160 = call "PlantillaTacteles2String.vi"("Plantilla_Tacteles"=w124) -> ("String_Tácteles"=w123:string)  [unwired: 10 in]
                n161 = Bundle("Value"=w125, "String_Tácteles"=w123, "Number of Rows"=w122, "Number of Columns"=w119, "Value"=w121, "Value"=w120, "Value"=w117) -> (w118:T6)  [unwired: 1 in]
                n162 = call "Guardado_Sesion.vi"("Guardar_Sesion"=w118) -> ("Menu_Ring_String"=w126:string[])  [unwired: 10 in]
                n163 = property on="Sesiones Disponibles" class="Ring (strict)"("Strings []"=w126) -> ()  [unwired: 2 in, 2 out]
              }
              frame True {
                n164 = One Button Dialog(message="Por favor, introduzca un nombre\npara esta sesión antes de pulsar el\nbotón Guardar.") -> ()  [unwired: 1 in, 1 out]
              }
            }
          }
          event "OK_Manual": Value Change {
            w130 = TRUE ("Visible")
            n165 = event-data() -> ()  [unwired: 1 in, 6 out]
            n166 = property on="NºFilas" class="DigNum (strict)"() -> ("Value"=w137:i32)  [unwired: 2 in, 2 out]
            n167 = property on="Nº Columnas" class="DigNum (strict)"() -> ("Value"=w136:i32)  [unwired: 2 in, 2 out]
            n168 = property on="Tab_Valvula" class="TabCtl (strict)"("Visible"=w130) -> ()  [unwired: 2 in, 2 out]
            n169 = property on="Selección Modo Datos" class="Enum (strict)"("Visible"=w130) -> ()  [unwired: 2 in, 2 out]
            n170 = property on="Tab_Introducción_Datos" class="TabCtl (strict)"("Visible"=w130) -> ()  [unwired: 2 in, 2 out]
            n171 = property on="Intensity Graph" class="IntGraph (strict)"("Visible"=w130) -> ()  [unwired: 2 in, 2 out]
            n172 = property on="XY Graph" class="XYGraph (strict)"("Visible"=w130) -> ()  [unwired: 2 in, 2 out]
            n173 = property on="Fila" class="DigNum (strict)"("Visible"=w130) -> ()  [unwired: 2 in, 2 out]
            n174 = property on="Columna" class="DigNum (strict)"("Visible"=w130) -> ()  [unwired: 2 in, 2 out]
            n175 = property on="Plantilla Tácteles" class="Arr (strict)"("Number of Rows"=w137) -> ()  [unwired: 2 in, 2 out]
            n176 = property on="Save Button" class="Bool (strict)"("DisabledEnum"=T3."Enabled" ("Disabled")) -> ()  [unwired: 2 in, 2 out]
            n177 = property on="Nombre Nueva Sesión" class="Str"("DisabledEnum"=T3."Enabled" ("Disabled")) -> ()  [unwired: 2 in, 2 out]
            n178 = property on="Plantilla Tácteles" class="Arr (strict)"("Number of Columns"=w136) -> ()  [unwired: 2 in, 2 out]
            n179 = property on="Fila" class="DigNum (strict)"("Visible"=w130) -> ()  [unwired: 2 in, 2 out]
            n180 = property on="Columna" class="DigNum (strict)"("Visible"=w130) -> ()  [unwired: 2 in, 2 out]
            n181 = property on="Nombre .csv" class="Str"("Visible"=w130) -> ()  [unwired: 2 in, 2 out]
            n182 = property on="Export Button" class="Bool (strict)"("Visible"=w130) -> ()  [unwired: 2 in, 2 out]
            n183 = property on="Valor_Maximo" class="DigNum (strict)"() -> ("Value"=w128:i32)  [unwired: 2 in, 2 out]
            n184 = property on="Plantilla Tácteles" class="Arr (strict)"() -> ("Number of Columns"=w133:u32, "Number of Rows"=w134:u32)  [unwired: 2 in, 2 out]
            n185 = property on="Ejecutar Válvula" class="Bool (strict)"("DisabledEnum"=T3."Enabled" ("Disabled")) -> ()  [unwired: 2 in, 2 out]
            n186 = property on="Intensity Graph" class="IntGraph (strict)"("ZScale.Maximum"=w128) -> ()  [unwired: 2 in, 2 out]
            n187 = property on="XY Graph" class="XYGraph (strict)"("YScale.Maximum"=w128) -> ()  [unwired: 2 in, 2 out]
            n188 = property on="Intensity Graph" class="IntGraph (strict)"("Transpose Array"=TRUE) -> ()  [unwired: 2 in, 2 out]
            n189 = property on="Intensity Graph" class="IntGraph (strict)"("YScale.Maximum"=w134) -> ()  [unwired: 2 in, 2 out]
            n190 = property on="Intensity Graph" class="IntGraph (strict)"("XScale.Maximum"=w133) -> ()  [unwired: 2 in, 2 out]
          }
          event "Home Button": Value Change {
            w143 = FALSE ("Manual")
            w145 = 0
            w147 = TRUE ("Visible")
            w140 = FALSE ("Visible")
            n191 = event-data() -> ()  [unwired: 1 in, 6 out]
            n192 = property on="Home Button" class="Bool (strict)"("Visible"=w140) -> ()  [unwired: 2 in, 2 out]
            n193 = property on="Save Button" class="Bool (strict)"("Visible"=w140) -> ()  [unwired: 2 in, 2 out]
            n194 = property on="Refresh Button" class="Bool (strict)"("Visible"=w140) -> ()  [unwired: 2 in, 2 out]
            n195 = property on="Sesiones Disponibles" class="Ring (strict)"("Visible"=w140) -> ()  [unwired: 2 in, 2 out]
            n196 = property on="Tab Control" class="TabCtl (strict)"("Visible"=w140) -> ()  [unwired: 2 in, 2 out]
            n197 = property on="Automática" class="Bool (strict)"("Visible"=w140) -> ()  [unwired: 2 in, 2 out]
            n198 = property on="Nombre Nueva Sesión" class="Str"("Visible"=w140) -> ()  [unwired: 2 in, 2 out]
            n199 = property on="Manual" class="Bool (strict)"("Visible"=w140) -> ()  [unwired: 2 in, 2 out]
            n200 = property on="Tab_Introducción_Datos" class="TabCtl (strict)"("Visible"=w140) -> ()  [unwired: 2 in, 2 out]
            n201 = property on="Selección Modo Datos" class="Enum (strict)"("Visible"=w140) -> ()  [unwired: 2 in, 2 out]
            n202 = property on="Tab Control" class="TabCtl (strict)"("Tabs Visible?"=w140) -> ()  [unwired: 2 in, 2 out]
            n203 = property on="Open Button" class="Bool (strict)"("Visible"=w147) -> ()  [unwired: 2 in, 2 out]
            n204 = property on="Settings Button" class="Bool (strict)"("Visible"=w147) -> ()  [unwired: 2 in, 2 out]
            n205 = property on="Automática" class="Bool (strict)"("Value"=FALSE ("Automática")) -> ()  [unwired: 2 in, 2 out]
            n206 = property on="Manual" class="Bool (strict)"("Value"=w143) -> ()  [unwired: 2 in, 2 out]
            n207 = property on="Tab_Valvula" class="TabCtl (strict)"("Visible"=w143) -> ()  [unwired: 2 in, 2 out]
            n208 = property on="Plantilla Tácteles" class="Arr (strict)"("Number of Rows"=w145) -> ()  [unwired: 2 in, 2 out]
            n209 = property on="Plantilla Tácteles" class="Arr (strict)"("Number of Columns"=w145) -> ()  [unwired: 2 in, 2 out]
            n210 = property on="Plantilla Tácteles" class="Arr (strict)"("Value"=bool[][] [[FALSE]]) -> ()  [unwired: 2 in, 2 out]
          }
          event "Selección Modo Datos": Value Change {
            n211 = event-data() -> ()  [unwired: 1 in, 6 out]
            n212 = property on="Selección Modo Datos" class="Enum (strict)"() -> ("Value"=w150:T1)  [unwired: 2 in, 2 out]
            n213 = case shown="\"Manual\", Default" w150 {
              frame "Manual", Default {
                n214 = property on="Tab_Introducción_Datos" class="TabCtl (strict)"("Value"=T2."Manual" ("Tab_Introducción_Datos")) -> ()  [unwired: 2 in, 2 out]
              }
              frame "Puerto Serie" {
                n215 = property on="Tab_Introducción_Datos" class="TabCtl (strict)"("Value"=T2."Puerto Serie" ("Tab_Introducción_Datos")) -> ()  [unwired: 2 in, 2 out]
              }
              frame "Archivo Importado" {
                n216 = property on="Tab_Introducción_Datos" class="TabCtl (strict)"("Value"=T2."Archivo Importado" ("Tab_Introducción_Datos")) -> ()  [unwired: 2 in, 2 out]
              }
            }
          }
          event "Comando Manual": Mouse Down {
            n217 = event-data() -> ()  [unwired: 1 in, 8 out]
            n218 = Unbundle(w175) -> (w174:dbl[][][], w173:dbl[])
            n219 = property on="Cadena de datos (Manual)" class="Str"() -> ("Value"=w160:string)  [unwired: 2 in, 2 out]
            n220 = property on="Plantilla Tácteles" class="Arr (strict)"() -> ("Value"=w178:bool[][], "Number of Rows"=w177:u32, "Number of Columns"=w176:u32)  [unwired: 2 in, 2 out]
            n221 = property on="Proporcional" class="DigNum (strict)"() -> ("Value"=w157:i32)  [unwired: 2 in, 2 out]
            n222 = property on="N_Bits" class="DigNum (strict)"() -> ("Value"=w158:i32)  [unwired: 2 in, 2 out]
            n223 = Number To Boolean Array(number=w157) -> (Boolean array=w156:bool[])
            n224 = Index Array(array=w156, index=0) -> (element=w154:bool)
            n225 = call "Inversión_Cuenta.vi"("Activador"=w154, "Datos_Sensores_In"=w160, "N_Bits"=w158) -> ("Datos_Sensores_Out"=w159:string)  [unwired: 8 in]
            n226 = property on="Presión Manual(PSI)" class="DigNum (strict)"() -> ("Value"=w172:dbl)  [unwired: 2 in, 2 out]
            n227 = call "Construye_Matriz_Tacteles_2D (SubVI).vi"("Datos string"=w159, "Plantilla Tácteles"=w178, "Columnas"=w176, "Filas"=w177) -> ("Valores Tácteles"=w170:dbl[][])  [unwired: 6 in, 1 out]
            "Valores Tácteles" <- w170
            n228 = property on="Fila" class="DigNum (strict)"() -> ("Value"=w165:i32)  [unwired: 2 in, 2 out]
            n229 = property on="Columna" class="DigNum (strict)"() -> ("Value"=w164:i32)  [unwired: 2 in, 2 out]
            n230 = Build Array (concatenate)(w173, w172) -> (w168:dbl[])
            n231 = Build Array (concatenate)(w174, w170) -> (w166:dbl[][][])
            n232 = property on="Intensity Graph" class="IntGraph (strict)"("Value"=w170) -> ()  [unwired: 2 in, 2 out]
            n233 = Bundle(w166, w168) -> (w171:cluster{dbl[][][], dbl[]})  [unwired: 1 in]
            n234 = Index Array(array=w166, index (dim 1)=w165, index (dim 2)=w164) -> (element=w163:dbl[])  [unwired: 1 in]
            n235 = call "Convert to Dynamic Data"("Array"=w168) -> ("Dynamic Data Type"=w167:dynamicdata)  [unwired: 3 in]
            n236 = call "Convert to Dynamic Data2"("Array"=w163) -> ("Dynamic Data Type"=w162:dynamicdata)  [unwired: 3 in]
            n237 = call "Build XY Graph"("Y Input"=w162, "X Input"=w167) -> ("XY Graph"=w169:cluster{"X":dbl[], "Y":dbl[]}[])  [unwired: 8 in, 1 out]
            n238 = property on="XY Graph" class="XYGraph (strict)"("Value"=w169) -> ()  [unwired: 2 in, 2 out]
          }
          event "Recibir de fichero": Mouse Down {
            n239 = event-data() -> ()  [unwired: 1 in, 8 out]
            n240 = property on="Proporcional" class="DigNum (strict)"() -> ("Value"=w184:i32)  [unwired: 2 in, 2 out]
            n241 = Unbundle(w205) -> (w203:dbl[][][], w202:dbl[])
            n242 = property on="file path (use dialog)" class="Path"() -> ("Value"=w206:path)  [unwired: 2 in, 2 out]
            n243 = Number To Boolean Array(number=w184) -> (Boolean array=w183:bool[])
            n244 = Index Array(array=w183, index=0) -> (element=w180:bool)
            n245 = call "Import_txt.vi"("i in"=w188, "Mandar Comando"=TRUE, "file path (use dialog)"=w206) -> ("i out"=w187:i32, "Presión (PSI)"=w204:dbl, "Medicion"=w185:string)  [unwired: 5 in, 1 out]
            n246 = property on="N_Bits" class="DigNum (strict)"() -> ("Value"=w181:i32)  [unwired: 2 in, 2 out]
            n247 = call "Inversión_Cuenta.vi"("Activador"=w180, "Datos_Sensores_In"=w185, "N_Bits"=w181) -> ("Datos_Sensores_Out"=w179:string)  [unwired: 8 in]
            n248 = property on="Plantilla Tácteles" class="Arr (strict)"() -> ("Value"=w200:bool[][], "Number of Rows"=w201:u32, "Number of Columns"=w199:u32)  [unwired: 2 in, 2 out]
            n249 = Build Array (concatenate)(w202, w204) -> (w196:dbl[])
            n250 = call "Construye_Matriz_Tacteles_2D (SubVI).vi"("Datos string"=w179, "Plantilla Tácteles"=w200, "Columnas"=w199, "Filas"=w201) -> ("Valores Tácteles"=w197:dbl[][])  [unwired: 6 in, 1 out]
            n251 = Build Array (concatenate)(w203, w197) -> (w194:dbl[][][])
            n252 = property on="Fila" class="DigNum (strict)"() -> ("Value"=w192:i32)  [unwired: 2 in, 2 out]
            n253 = property on="Columna" class="DigNum (strict)"() -> ("Value"=w193:i32)  [unwired: 2 in, 2 out]
            n254 = property on="Intensity Graph" class="IntGraph (strict)"("Value"=w197) -> ()  [unwired: 2 in, 2 out]
            n255 = Index Array(array=w194, index (dim 1)=w192, index (dim 2)=w193) -> (element=w191:dbl[])  [unwired: 1 in]
            n256 = Bundle(w194, w196) -> (w189:cluster{dbl[][][], dbl[]})  [unwired: 1 in]
            n257 = call "Convert to Dynamic Data11"("Array"=w196) -> ("Dynamic Data Type"=w195:dynamicdata)  [unwired: 3 in]
            n258 = call "Convert to Dynamic Data12"("Array"=w191) -> ("Dynamic Data Type"=w190:dynamicdata)  [unwired: 3 in]
            n259 = call "Build XY Graph6"("Y Input"=w190, "X Input"=w195) -> ("XY Graph"=w198:cluster{"X":dbl[], "Y":dbl[]}[])  [unwired: 8 in, 1 out]
            n260 = property on="XY Graph" class="XYGraph (strict)"("Value"=w198) -> ()  [unwired: 2 in, 2 out]
          }
          event "Medida Simple": Mouse Down {
            n261 = event-data() -> ()  [unwired: 1 in, 8 out]
            n262 = property on="COM PSoC" class="VISAName"() -> ("Value"=w220:refnum<visa-resource-name>)  [unwired: 2 in, 2 out]
            n263 = property on="baud rate PSoC" class="Ring (strict)"() -> ("Value"=w219:u32)  [unwired: 2 in, 2 out]
            n264 = call "Comunicación_PSoC_con_Queue.vi"("write buffer"="R", "baud rate"=w219, "VISA resource name"=w220) -> ("UART Error"=w217:errorcluster, "unsigned byte array"=w207:u8[])  [unwired: 6 in, 1 out]
            n265 = property on="COM Pneumax" class="VISAName"() -> ("Value"=w222:refnum<visa-resource-name>)  [unwired: 2 in, 2 out]
            n266 = call "Uint16_2_String.vi"("unsigned byte array"=w207) -> ("String Formado"=w208:string)  [unwired: 9 in, 1 out]
            "Datos UART" <- w208
            n267 = Unbundle(w238) -> (w237:dbl[][][], w236:dbl[])
            n268 = property on="UART Error" class="Clust (strict)"("Value"=w217) -> ()  [unwired: 2 in, 2 out]
            n269 = call "RegCommands_Mod.vi"("VISA resource name"=w222, "Command Type"="Reading outlet pressure value") -> ("Regulator answer"=w221:string, "Pressure (PSI)"=w235:dbl)  [unwired: 8 in]
            n270 = property on="Proporcional" class="DigNum (strict)"() -> ("Value"=w213:i32)  [unwired: 2 in, 2 out]
            n271 = property on="Respuesta del regulador" class="Str"("Value"=w221) -> ()  [unwired: 2 in, 2 out]
            n272 = Number To Boolean Array(number=w213) -> (Boolean array=w214:bool[])
            n273 = property on="Plantilla Tácteles" class="Arr (strict)"() -> ("Value"=w224:bool[][], "Number of Rows"=w225:u32, "Number of Columns"=w226:u32)  [unwired: 2 in, 2 out]
            n274 = property on="N_Bits" class="DigNum (strict)"() -> ("Value"=w210:i32)  [unwired: 2 in, 2 out]
            n275 = Index Array(array=w214, index=0) -> (element=w209:bool)
            n276 = call "Inversión_Cuenta.vi"("Activador"=w209, "Datos_Sensores_In"=w208, "N_Bits"=w210) -> ("Datos_Sensores_Out"=w211:string)  [unwired: 8 in]
            n277 = Build Array (concatenate)(w236, w235) -> (w229:dbl[])
            n278 = call "Construye_Matriz_Tacteles_2D (SubVI).vi"("Datos string"=w211, "Plantilla Tácteles"=w224, "Columnas"=w226, "Filas"=w225) -> ("Valores Tácteles"=w216:dbl[][])  [unwired: 6 in, 1 out]
            n279 = Build Array (concatenate)(w237, w216) -> (w234:dbl[][][])
            n280 = property on="Valores Tácteles" class="Arr (strict)"("Value"=w216) -> ()  [unwired: 2 in, 2 out]
            n281 = property on="Columna" class="DigNum (strict)"() -> ("Value"=w233:i32)  [unwired: 2 in, 2 out]
            n282 = property on="Fila" class="DigNum (strict)"() -> ("Value"=w232:i32)  [unwired: 2 in, 2 out]
            n283 = property on="Intensity Graph" class="IntGraph (strict)"("Value"=w216) -> ()  [unwired: 2 in, 2 out]
            n284 = Index Array(array=w234, index (dim 1)=w232, index (dim 2)=w233) -> (element=w231:dbl[])  [unwired: 1 in]
            n285 = Bundle(w234, w229) -> (w223:cluster{dbl[][][], dbl[]})  [unwired: 1 in]
            n286 = call "Convert to Dynamic Data3"("Array"=w231) -> ("Dynamic Data Type"=w230:dynamicdata)  [unwired: 3 in]
            n287 = call "Convert to Dynamic Data4"("Array"=w229) -> ("Dynamic Data Type"=w228:dynamicdata)  [unwired: 3 in]
            n288 = call "Build XY Graph2"("Y Input"=w230, "X Input"=w228) -> ("XY Graph"=w227:cluster{"X":dbl[], "Y":dbl[]}[])  [unwired: 8 in, 1 out]
            n289 = property on="XY Graph" class="XYGraph (strict)"("Value"=w227) -> ()  [unwired: 2 in, 2 out]
          }
          event "Deriva": Mouse Down {
            n290 = event-data() -> ()  [unwired: 1 in, 8 out]
            n291 = flat-sequence {
              tunnel: [w264] -> w242
              tunnel: [w263] -> w241
              frame #0 {
                w249 = T3."Disabled and Grayed Out" ("Disabled")
                n292 = property on="Medida Simple" class="Bool (strict)"("DisabledEnum"=w249) -> ()  [unwired: 2 in, 2 out]
                n293 = property on="Comando Manual" class="Bool (strict)"("DisabledEnum"=w249) -> ()  [unwired: 2 in, 2 out]
                n294 = property on="Histéresis" class="Bool (strict)"("DisabledEnum"=w249) -> ()  [unwired: 2 in, 2 out]
              }
              frame #1 {
                n295 = property on="Tiempo Entre Medida(ms)" class="DigNum (strict)"() -> ("Value"=w268:dbl)  [unwired: 2 in, 2 out]
                n296 = property on="Tiempo Total" class="DigNum (strict)"() -> ("Value"=w269:dbl)  [unwired: 2 in, 2 out]
                n297 = Divide(x=w269, y=w268) -> (x/y=w252:dbl)
                n298 = Decrement(x=w252) -> (x-1=w251:dbl)
                n299 = for {
                  N: w251 -> [_]
                  tunnel: w268 -> [w273]
                  tunnel: [w272] -> w263 mode=indexing
                  tunnel: [w271] -> w250 mode=indexing
                  n300 = flat-sequence {
                    tunnel: [w274] -> w272
                    tunnel: [w285] -> w271
                    frame #0 {
                      n301 = property on="Presión Deseada (PSI)" class="DigNum (strict)"() -> ("Value"=w277:dbl)  [unwired: 2 in, 2 out]
                      n302 = call "RegCommands_Mod.vi"("Desired pressure (PSI)"=w277, "Command Type"="Setting the desired pressure") -> ("Regulator answer"=w275:string, "Pressure (PSI)"=w274:dbl)  [unwired: 8 in]
                      n303 = property on="Respuesta del regulador" class="Str"("Value"=w275) -> ()  [unwired: 2 in, 2 out]
                      n304 = property on="Presión (PSI)" class="DigNum (strict)"("Value"=w274) -> ()  [unwired: 2 in, 2 out]
                    }
                    frame #1 {
                      n305 = property on="COM PSoC" class="VISAName"() -> ("Value"=w289:refnum<visa-resource-name>)  [unwired: 2 in, 2 out]
                      n306 = property on="baud rate PSoC" class="Ring (strict)"() -> ("Value"=w288:u32)  [unwired: 2 in, 2 out]
                      n307 = property on="Proporcional" class="DigNum (strict)"() -> ("Value"=w283:i32)  [unwired: 2 in, 2 out]
                      n308 = call "Comunicación_PSoC_con_Queue.vi"("write buffer"="R", "baud rate"=w288, "VISA resource name"=w289) -> ("UART Error"=w286:errorcluster, "unsigned byte array"=w279:u8[])  [unwired: 6 in, 1 out]
                      n309 = property on="UART Error" class="Clust (strict)"("Value"=w286) -> ()  [unwired: 2 in, 2 out]
                      n310 = property on="N_Bits" class="DigNum (strict)"() -> ("Value"=w284:i32)  [unwired: 2 in, 2 out]
                      n311 = Number To Boolean Array(number=w283) -> (Boolean array=w282:bool[])
                      n312 = call "Uint16_2_String.vi"("unsigned byte array"=w279) -> ("String Formado"=w278:string)  [unwired: 9 in, 1 out]
                      n313 = Index Array(array=w282, index=0) -> (element=w280:bool)
                      n314 = call "Inversión_Cuenta.vi"("Activador"=w280, "Datos_Sensores_In"=w278, "N_Bits"=w284) -> ("Datos_Sensores_Out"=w285:string)  [unwired: 8 in]
                    }
                  }
                  n315 = Wait (ms)(milliseconds to wait=w273) -> ()  [unwired: 1 out]
                }
                n316 = property on="Plantilla Tácteles" class="Arr (strict)"() -> ("Value"=w255:bool[][], "Number of Rows"=w254:u32, "Number of Columns"=w253:u32)  [unwired: 2 in, 2 out]
                n317 = call "Construye_Matriz_Tacteles(SubVI).vi"("Filas"=w254, "Columnas"=w253, "Plantilla Tácteles"=w255, "String Array Datos"=w250) -> ("Array 3D"=w264:dbl[][][])  [unwired: 3 in, 2 out]
                n318 = property on="Fila" class="DigNum (strict)"() -> ("Value"=w261:i32)  [unwired: 2 in, 2 out]
                n319 = property on="Columna" class="DigNum (strict)"() -> ("Value"=w260:i32)  [unwired: 2 in, 2 out]
                n320 = Array Size(array=w264) -> (size(s)=w266:i32[])
                n321 = Index Array(array=w266, index=0) -> (element=w265:i32)
                n322 = Index Array(array=w264, index (dim 1)=w261, index (dim 2)=w260) -> (element=w259:dbl[])  [unwired: 1 in]
                n323 = call "Promediado_Tacteles.vi"("Activador"=TRUE, "Muestras Promedio"=w265, "3D Tácteles"=w264) -> ("Matriz promediada"=w256:dbl[][])  [unwired: 8 in]
                n324 = call "Convert to Dynamic Data5"("Array"=w263) -> ("Dynamic Data Type"=w262:dynamicdata)  [unwired: 3 in]
                n325 = call "Convert to Dynamic Data6"("Array"=w259) -> ("Dynamic Data Type"=w258:dynamicdata)  [unwired: 3 in]
                n326 = property on="Intensity Graph" class="IntGraph (strict)"("Value"=w256) -> ()  [unwired: 2 in, 2 out]
                n327 = call "Build XY Graph3"("Y Input"=w258, "X Input"=w262) -> ("XY Graph"=w257:cluster{"X":dbl[], "Y":dbl[]}[])  [unwired: 8 in, 1 out]
                n328 = property on="XY Graph" class="XYGraph (strict)"("Value"=w257) -> ()  [unwired: 2 in, 2 out]
              }
              frame #2 {
                w290 = T3."Enabled" ("Disabled")
                n329 = property on="Comando Manual" class="Bool (strict)"("DisabledEnum"=w290) -> ()  [unwired: 2 in, 2 out]
                n330 = property on="Medida Simple" class="Bool (strict)"("DisabledEnum"=w290) -> ()  [unwired: 2 in, 2 out]
                n331 = property on="Histéresis" class="Bool (strict)"("DisabledEnum"=w290) -> ()  [unwired: 2 in, 2 out]
              }
            }
            n332 = Unbundle(w248) -> (w246:dbl[][][], w247:dbl[])
            n333 = Insert Into Array(array=w247, new element=w241) -> (w245:dbl[])  [unwired: 1 in]
            n334 = Insert Into Array(array=w246, new element=w242) -> (w244:dbl[][][])  [unwired: 3 in]
            n335 = Bundle(w244, w245) -> (w243:cluster{dbl[][][], dbl[]})  [unwired: 1 in]
          }
          event "Histéresis": Mouse Down {
            n336 = event-data() -> ()  [unwired: 1 in, 8 out]
            n337 = flat-sequence {
              tunnel: w295 -> [w297]
              tunnel: [w297] -> w294
              tunnel: w294 -> [w301]
              tunnel: [w300] -> w293
              tunnel: w293 -> [w363]
              tunnel: [w363] -> w292
              frame #0 {
                w296 = T3."Disabled and Grayed Out" ("Disabled")
                n338 = property on="Medida Simple" class="Bool (strict)"("DisabledEnum"=w296) -> ()  [unwired: 2 in, 2 out]
                n339 = property on="Deriva" class="Bool (strict)"("DisabledEnum"=w296) -> ()  [unwired: 2 in, 2 out]
                n340 = property on="Comando Manual" class="Bool (strict)"("DisabledEnum"=w296) -> ()  [unwired: 2 in, 2 out]
              }
              frame #1 {
                n341 = property on="COM Pneumax" class="VISAName"() -> ("Value"=w305:refnum<visa-resource-name>)  [unwired: 2 in, 2 out]
                n342 = property on="N_Bits" class="DigNum (strict)"() -> ("Value"=w299:i32)  [unwired: 2 in, 2 out]
                n343 = property on="Proporcional" class="DigNum (strict)"() -> ("Value"=w298:i32)  [unwired: 2 in, 2 out]
                n344 = property on="Nº De Ejecuciones" class="DigNum (strict)"() -> ("Value"=w303:dbl)  [unwired: 2 in, 2 out]
                n345 = property on="COM PSoC" class="VISAName"() -> ("Value"=w306:refnum<visa-resource-name>)  [unwired: 2 in, 2 out]
                n346 = property on="baud rate PSoC" class="Ring (strict)"() -> ("Value"=w307:u32)  [unwired: 2 in, 2 out]
                n347 = Decrement(x=w303) -> (x-1=w302:dbl)
                n348 = Bundle("Value"=w306, "Value"=w307, "Value"=w305, "Value"=w299, "Value"=w298) -> (w304:T7)  [unwired: 1 in]
                n349 = for {
                  N: w302 -> [_]
                  tunnel: w304 -> [w341]
                  shift-right: [w308] -> w300
                  shift-left: w301 -> [w315]
                  n350 = property on="Tiempo Entre Medidas(ms)" class="DigNum (strict)"() -> ("Value"=w327:dbl)  [unwired: 2 in, 2 out]
                  n351 = property on="Presión Min (PSI)" class="DigNum (strict)"() -> ("Value"=w331:dbl)  [unwired: 2 in, 2 out]
                  n352 = property on="Incremento" class="DigNum (strict)"() -> ("Value"=w332:dbl)  [unwired: 2 in, 2 out]
                  n353 = property on="Presión Max (PSI)" class="DigNum (strict)"() -> ("Value"=w330:dbl)  [unwired: 2 in, 2 out]
                  n354 = flat-sequence {
                    tunnel: w341 -> [w351]
                    tunnel: [w348] -> w337
                    tunnel: [w347] -> w339
                    tunnel: w330 -> [w346]
                    tunnel: w332 -> [w345]
                    tunnel: w331 -> [w344]
                    tunnel: [w345] -> w329
                    tunnel: [w344] -> w328
                    tunnel: w327 -> [w343]
                    tunnel: w341 -> [w361]
                    tunnel: [w358] -> w338
                    tunnel: [w357] -> w340
                    tunnel: w330 -> [w356]
                    tunnel: w329 -> [w355]
                    tunnel: w328 -> [w354]
                    tunnel: w327 -> [w353]
                    frame #0 {
                      n355 = call "Medida_Incremental.vi"("Activador"=TRUE, "Tiempo Entre Medidas (ms)"=w343, "Presión Min"=w344, "Presión Max"=w346, "Incremento"=w345, "Configuracion"=w351) -> ("UART Error"=w349:errorcluster, "Regulator answer"=w350:string, "Datos Array"=w348:string[], "Presión Array"=w347:dbl[])  [unwired: 2 in]
                      n356 = property on="Respuesta del regulador" class="Str"("Value"=w350) -> ()  [unwired: 2 in, 2 out]
                      n357 = property on="UART Error" class="Clust (strict)"("Value"=w349) -> ()  [unwired: 2 in, 2 out]
                    }
                    frame #1 {
                      n358 = call "Medida_Decremental(SubVI).vi"("Activador"=TRUE, "Tiempo Entre Medidas"=w353, "Presión Min"=w354, "Decremento"=w355, "Presión Max"=w356, "Configuracion"=w361) -> ("UART Error"=w359:errorcluster, "Regulator answer"=w360:string, "Presión Array"=w357:dbl[], "Datos Array"=w358:string[])  [unwired: 2 in]
                      n359 = property on="Respuesta del regulador" class="Str"("Value"=w360) -> ()  [unwired: 2 in, 2 out]
                      n360 = property on="UART Error" class="Clust (strict)"("Value"=w359) -> ()  [unwired: 2 in, 2 out]
                    }
                  }
                  n361 = Unbundle(w315) -> (w313:dbl[][][], w314:dbl[])
                  n362 = property on="Plantilla Tácteles" class="Arr (strict)"() -> ("Value"=w335:bool[][], "Number of Rows"=w334:u32, "Number of Columns"=w333:u32)  [unwired: 2 in, 2 out]
                  n363 = Insert Into Array(array=w339, new element=w340) -> (w312:dbl[])  [unwired: 1 in]
                  n364 = Insert Into Array(array=w337, new element=w338) -> (w336:string[])  [unwired: 1 in]
                  n365 = call "Construye_Matriz_Tacteles(SubVI).vi"("Filas"=w334, "Columnas"=w333, "Plantilla Tácteles"=w335, "String Array Datos"=w336) -> ("Array 3D"=w311:dbl[][][])  [unwired: 3 in, 2 out]
                  n366 = Array Size(array=w311) -> (size(s)=w325:i32[])
                  n367 = property on="Fila" class="DigNum (strict)"() -> ("Value"=w319:i32)  [unwired: 2 in, 2 out]
                  n368 = property on="Columna" class="DigNum (strict)"() -> ("Value"=w318:i32)  [unwired: 2 in, 2 out]
                  n369 = Insert Into Array(array=w313, new element=w311) -> (w310:dbl[][][])  [unwired: 3 in]
                  n370 = Insert Into Array(array=w314, new element=w312) -> (w309:dbl[])  [unwired: 1 in]
                  n371 = Index Array(array=w325, index=0) -> (element=w324:i32)
                  n372 = Index Array(array=w311, index (dim 1)=w319, index (dim 2)=w318) -> (element=w317:dbl[])  [unwired: 1 in]
                  n373 = Bundle(w310, w309) -> (w308:cluster{dbl[][][], dbl[]})  [unwired: 1 in]
                  n374 = call "Promediado_Tacteles.vi"("Activador"=TRUE, "Muestras Promedio"=w324, "3D Tácteles"=w311) -> ("Matriz promediada"=w322:dbl[][])  [unwired: 8 in]
                  n375 = call "Convert to Dynamic Data7"("Array"=w312) -> ("Dynamic Data Type"=w320:dynamicdata)  [unwired: 3 in]
                  n376 = call "Convert to Dynamic Data8"("Array"=w317) -> ("Dynamic Data Type"=w316:dynamicdata)  [unwired: 3 in]
                  n377 = property on="Intensity Graph" class="IntGraph (strict)"("Value"=w322) -> ()  [unwired: 2 in, 2 out]
                  n378 = call "Build XY Graph4"("Y Input"=w316, "X Input"=w320) -> ("XY Graph"=w321:cluster{"X":dbl[], "Y":dbl[]}[])  [unwired: 8 in, 1 out]
                  n379 = property on="XY Graph" class="XYGraph (strict)"("Value"=w321) -> ()  [unwired: 2 in, 2 out]
                }
              }
              frame #2 {
                w362 = T3."Enabled" ("Disabled")
                n380 = property on="Medida Simple" class="Bool (strict)"("DisabledEnum"=w362) -> ()  [unwired: 2 in, 2 out]
                n381 = property on="Deriva" class="Bool (strict)"("DisabledEnum"=w362) -> ()  [unwired: 2 in, 2 out]
                n382 = property on="Comando Manual" class="Bool (strict)"("DisabledEnum"=w362) -> ()  [unwired: 2 in, 2 out]
              }
            }
          }
          event "Export Button": Mouse Down {
            n383 = event-data() -> ()  [unwired: 1 in, 8 out]
            n384 = property on="Plantilla Tácteles" class="Arr (strict)"() -> ("Number of Rows"=w375:u32, "Number of Columns"=w374:u32)  [unwired: 2 in, 2 out]
            n385 = property on="Nombre .csv" class="Str"() -> ("Value"=w372:string)  [unwired: 2 in, 2 out]
            n386 = Current VI's Path() -> (path=w371:path)
            n387 = call "Crea_TXT.vi"("Activador"=TRUE, "VI path"=w371, "Columnas"=w374, "Filas"=w375, "IN_Datos"=w366, "Nombre  .txt"=w372) -> ()  [unwired: 6 in]
            n388 = Two Button Dialog(message="Datos Exportados. ¿Desea borrar la base de datos?", 1:"No" ("F button name (\"Cancel\")"), 2:"Sí" ("T button name (\"OK\")")) -> (T button?=w370:bool)
            n389 = case shown="False" w370 {
              tunnel: w366 -> [w376 _]
              tunnel: [w376 cluster{dbl[][][], dbl[]} {[], []}] -> w365
              frame False {
              }
              frame True {
              }
            }
          }
          event "Fila", "Columna": Value Change {
            w381 = dbl[] []
            # "Borra los datos de la gráfica en caso de que se selecciones otro táctel diferente.\nEvitando que se mezclen datos de distintos tacteles."
            n390 = event-data() -> ()  [unwired: 1 in, 6 out]
            n391 = call "Convert to Dynamic Data9"("Array"=w381) -> ("Dynamic Data Type"=w382:dynamicdata)  [unwired: 3 in]
            n392 = call "Convert to Dynamic Data10"("Array"=w381) -> ("Dynamic Data Type"=w380:dynamicdata)  [unwired: 3 in]
            n393 = call "Build XY Graph5"("Y Input"=w380, "X Input"=w382) -> ("XY Graph"=w379:cluster{"X":dbl[], "Y":dbl[]}[])  [unwired: 8 in, 1 out]
            n394 = property on="XY Graph" class="XYGraph (strict)"("Value"=w379) -> ()  [unwired: 2 in, 2 out]
          }
        }
      }
    }
    frame #2 {
      w383 = T3."Enabled" ("Disabled")
      w387 = TRUE ("Visible")
      w384 = TRUE ("Visible")
      n395 = property on="Home Button" class="Bool (strict)"("Visible"=w384) -> ()  [unwired: 2 in, 2 out]
      n396 = property on="Save Button" class="Bool (strict)"("Visible"=w384) -> ()  [unwired: 2 in, 2 out]
      n397 = property on="Refresh Button" class="Bool (strict)"("Visible"=w384) -> ()  [unwired: 2 in, 2 out]
      n398 = property on="Sesiones Disponibles" class="Ring (strict)"("Visible"=w384) -> ()  [unwired: 2 in, 2 out]
      n399 = property on="Automática" class="Bool (strict)"("Visible"=w384) -> ()  [unwired: 2 in, 2 out]
      n400 = property on="Manual" class="Bool (strict)"("Visible"=w384) -> ()  [unwired: 2 in, 2 out]
      n401 = property on="OK_Manual" class="Bool (strict)"("Visible"=w384) -> ()  [unwired: 2 in, 2 out]
      n402 = property on="OK_Automatico" class="Bool (strict)"("Visible"=w384) -> ()  [unwired: 2 in, 2 out]
      n403 = property on="Nombre Nueva Sesión" class="Str"("Visible"=w384) -> ()  [unwired: 2 in, 2 out]
      n404 = property on="Fila" class="DigNum (strict)"("Visible"=w384) -> ()  [unwired: 2 in, 2 out]
      n405 = property on="Tab Control" class="TabCtl (strict)"("Visible"=w384) -> ()  [unwired: 2 in, 2 out]
      n406 = property on="Columna" class="DigNum (strict)"("Visible"=w384) -> ()  [unwired: 2 in, 2 out]
      n407 = property on="Home Button" class="Bool (strict)"("Visible"=w384) -> ()  [unwired: 2 in, 2 out]
      n408 = property on="Tab_Valvula" class="TabCtl (strict)"("Visible"=w384) -> ()  [unwired: 2 in, 2 out]
      n409 = property on="Selección Modo Datos" class="Enum (strict)"("Visible"=w384) -> ()  [unwired: 2 in, 2 out]
      n410 = property on="Tab_Introducción_Datos" class="TabCtl (strict)"("Visible"=w384) -> ()  [unwired: 2 in, 2 out]
      n411 = property on="Intensity Graph" class="IntGraph (strict)"("Visible"=w384) -> ()  [unwired: 2 in, 2 out]
      n412 = property on="XY Graph" class="XYGraph (strict)"("Visible"=w384) -> ()  [unwired: 2 in, 2 out]
      n413 = property on="Plantilla Tácteles" class="Arr (strict)"("Number of Rows"=u32 0) -> ()  [unwired: 2 in, 2 out]
      n414 = property on="Settings Button" class="Bool (strict)"("Visible"=w387) -> ()  [unwired: 2 in, 2 out]
      n415 = property on="Plantilla Tácteles" class="Arr (strict)"("Number of Columns"=u32 0) -> ()  [unwired: 2 in, 2 out]
      n416 = property on="Comando Manual" class="Bool (strict)"("DisabledEnum"=w383) -> ()  [unwired: 2 in, 2 out]
      n417 = property on="Deriva" class="Bool (strict)"("DisabledEnum"=w383) -> ()  [unwired: 2 in, 2 out]
      n418 = property on="Open Button" class="Bool (strict)"("Visible"=w387) -> ()  [unwired: 2 in, 2 out]
      n419 = property on="Medida Simple" class="Bool (strict)"("DisabledEnum"=w383) -> ()  [unwired: 2 in, 2 out]
      n420 = property on="Histéresis" class="Bool (strict)"("DisabledEnum"=w383) -> ()  [unwired: 2 in, 2 out]
    }
  }
  n421 = disable-structure shown="Enabled" {
    frame Disabled {
      n422 = property on="Sesiones Disponibles" class="Ring (strict)"("Disabled Items []"=i32[] []) -> ()  [unwired: 2 in, 2 out]
      n423 = property on="COM Pneumax" class="VISAName" props=["Value"]() -> ()  [unwired: 2 in, 3 out]
    }
    frame Enabled {
    }
  }
